vi "Test.vi"() -> ()   [LabVIEW 2021]
uses:
  Commander/Commander.lvclass
  C:/Program Files (x86)/Hyper State Machine Framework/SSW_Hyper_State_Machine.lvlibp/State_Machine_Class/Main_State_Machine/Hyper_State_Machine.lvclass
  Common_State/Common_State.lvclass
  Image_Acquisition/Image_Acquisition.lvclass
  Motion_Control/Motion_Control.lvclass
  Data_Logging/Data_Logging.lvclass
  DIO/DIO.lvclass
  C:/Program Files (x86)/Hyper State Machine Framework/SSW_Hyper_State_Machine.lvlibp/State_Machine_Class/State_Machine_Module.llb/State Machine.ctl
  C:/Program Files (x86)/Hyper State Machine Framework/SSW_Hyper_State_Machine.lvlibp/State_Machine_Class/State_Machine_Module.llb/Lock_Unlock.ctl
  C:/Program Files (x86)/Hyper State Machine Framework/SSW_Hyper_State_Machine.lvlibp/State_Machine_Class/State_Machine_Module.llb/Iterval.ctl
  C:/Program Files (x86)/Hyper State Machine Framework/SSW_Hyper_State_Machine.lvlibp/State_Machine_Class/State_Machine_Module.llb/Time_Out.ctl
  <vilib>/numeric/Random Number (Range) DBL.vi
  <vilib>/Utility/High Resolution Relative Seconds.vi
  C:/Program Files (x86)/Hyper State Machine Framework/SSW_Hyper_State_Machine.lvlibp
panel:
  out "Activate":bool
  out "Lamp":bool
  out "Current_Pos":dbl caption="mm"
  in  "EMO":bool
  out "Product ID":string
  in  "Activate_Code(Blank for 30 min Trial)":string
  out "Heart_Rate":bool
  out "Heart rate(s)":dbl format="%#_6p"
  out "Execute rate(Hz)":dbl format="%#_6p"
  out "Base Class_Time_Act":bool
  out "Base Class_Elapsed Time(s)":dbl format="%#_6p"
  out "Base Class":bool=TRUE
  out "Base Class_Remaining(s)":dbl format="%#_6p"
  out "Base Class Progress":dbl(slide) scale=0.0..30.0
  in  "Base Class":dbl=30.0 max=1000.0 format="%#_13p"
  out "Base Class":string
  out "Base Class_Active":bool
  in  "Action Manager":T1(ring)
  out "Common":bool=TRUE
  out "Common_State":string
  out "Common_Time_Act":bool
  out "Common_Elapsed Time(s)":dbl format="%#_6p"
  out "Common_State Progress":dbl(slide) scale=0.0..3.0
  in  "Common_State_Interval":dbl=3.0 max=1000.0 format="%#_13p"
  out "Common_State_Active":bool
  out "Common_State_Remaining(s)":dbl format="%#_6p"
  out "Data Logging Progress":dbl(slide) scale=0.0..0.01
  out "DIO Progress":dbl(slide) scale=0.0..0.01
  out "Motion Control Progress":dbl(slide) scale=0.0..0.05
  out "Image Acquisition Progress":dbl(slide) scale=0.0..0.01
  out "Commander Progress":dbl(slide)=-1.0 scale=0.0..1.0
  out "Data_Logging":bool=TRUE
  out "Data Logging":string
  out "Data_Logging_Time_Act":bool
  out "Data_Logging_Elapsed Time(s)":dbl format="%#_6p"
  out "DIO":bool=TRUE
  out "DIO":string
  out "DIO_Time_Act":bool
  out "DIO_Elapsed Time(s)":dbl format="%#_6p"
  out "Motion_Control":bool=TRUE
  out "Motion_Control":string
  out "Motion_Control_Time_Act":bool
  out "Motion_Control_Elapsed Time(s)":dbl format="%#_6p"
  in  "Data Logging":dbl max=1000.0 format="%#_13p"
  out "Data Logging_Active":bool
  out "Data Logging_Remaining(s)":dbl format="%#_6p"
  in  "DIO_Interval":dbl=0.01 max=1000.0 format="%#_13p"
  in  "Motion_Control_Interval":dbl=0.05 max=1000.0 format="%#_13p"
  out "Motion Control_Act":bool
  out "DIO_Act":bool
  out "DIO_Remaining(s)":dbl format="%#_6p"
  out "Motion_Control_Remaining(s)":dbl format="%#_6p"
  in  "Image Acquisition_Interval":dbl=0.01 max=1000.0 format="%#_13p"
  in  "Commander_Interval":dbl max=1000.0 format="%#_13p"
  in  "System_Wait_Time":dbl=0.01 format="%#_13p"
  out "Commander_Active":bool
  out "Image Acquisition_Act":bool
  out "Image Acquisition_Remaining(s)":dbl format="%#_6p"
  out "Commander_Remaining(s)":dbl format="%#_6p"
  out "Image Acquisition":bool=TRUE
  out "Image Acquisition":string
  out "Commander":bool=TRUE
  out "Image Acquisition_Time_Act":bool
  out "Image Acquisition_Elapsed Time(s)":dbl format="%#_6p"
  out "Commander":string
  out "State1_Time_Act":bool
  out "Commander_Elapsed Time(s)":dbl format="%#_6p"
  in  "Stop":bool
  # "Note : Each State is Waiting Until Commader State Finished on \"Interval_Delay\" and then Unlock"
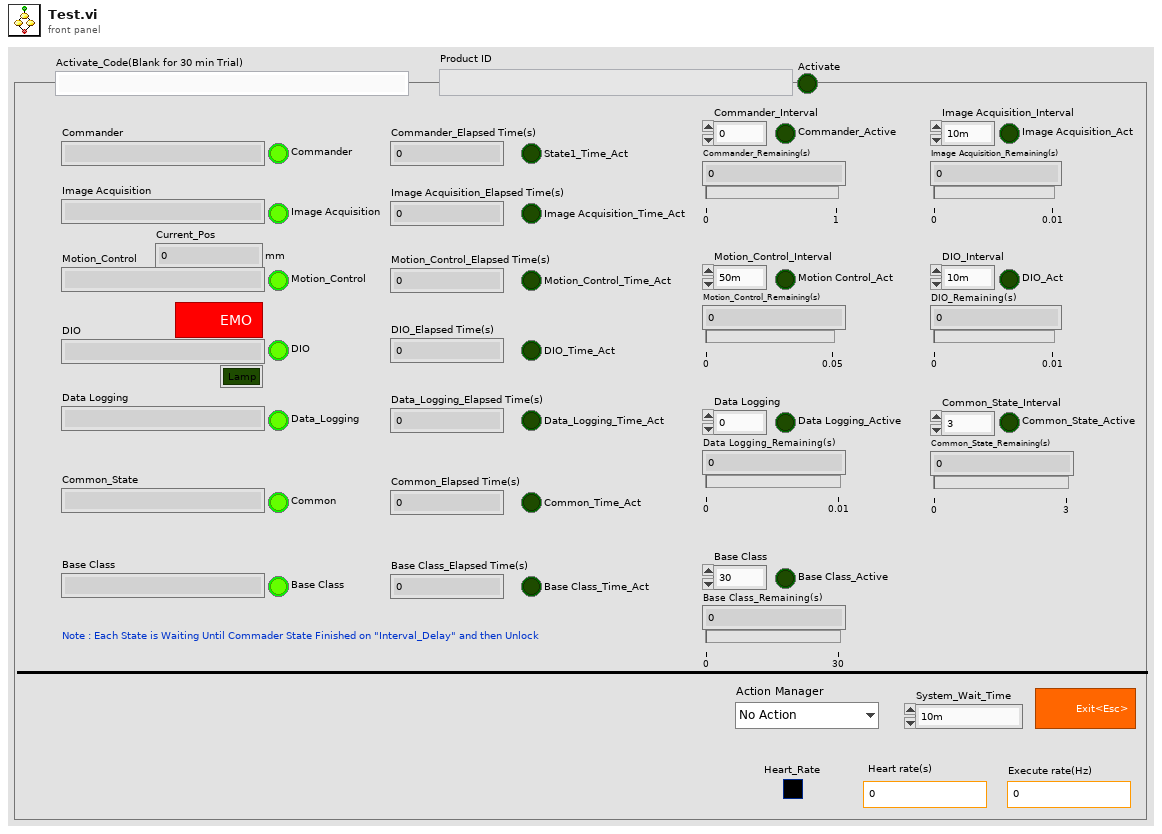
[diagram p1: front panel]
types:
  T1 = enum16{"No Action", "Init", "Lock", "Unlock", "Release"}
  T2 = typedef "SSW_Hyper_State_Machine.lvlibp/State Machine.ctl" = cluster{"Command":string, "Data":variant}
  T3 = typedef "SSW_Hyper_State_Machine.lvlibp/Time_Out.ctl" = cluster{"Enable(True)":bool, "Time Out_State Name":string, "Time Target (1s)":dbl, "Time Out_Reply Message_State":string}
  T4 = typedef "SSW_Hyper_State_Machine.lvlibp/Lock_Unlock.ctl" = cluster{"Action_Mode (Get)":enum16{"Set", "Get"}, "Action_Set (False)":bool, "State_In (Wait)":string}
  T5 = typedef "SSW_Hyper_State_Machine.lvlibp/Iterval.ctl" = cluster{"Delay(s)":dbl, "State (Interval_Delay)":string}
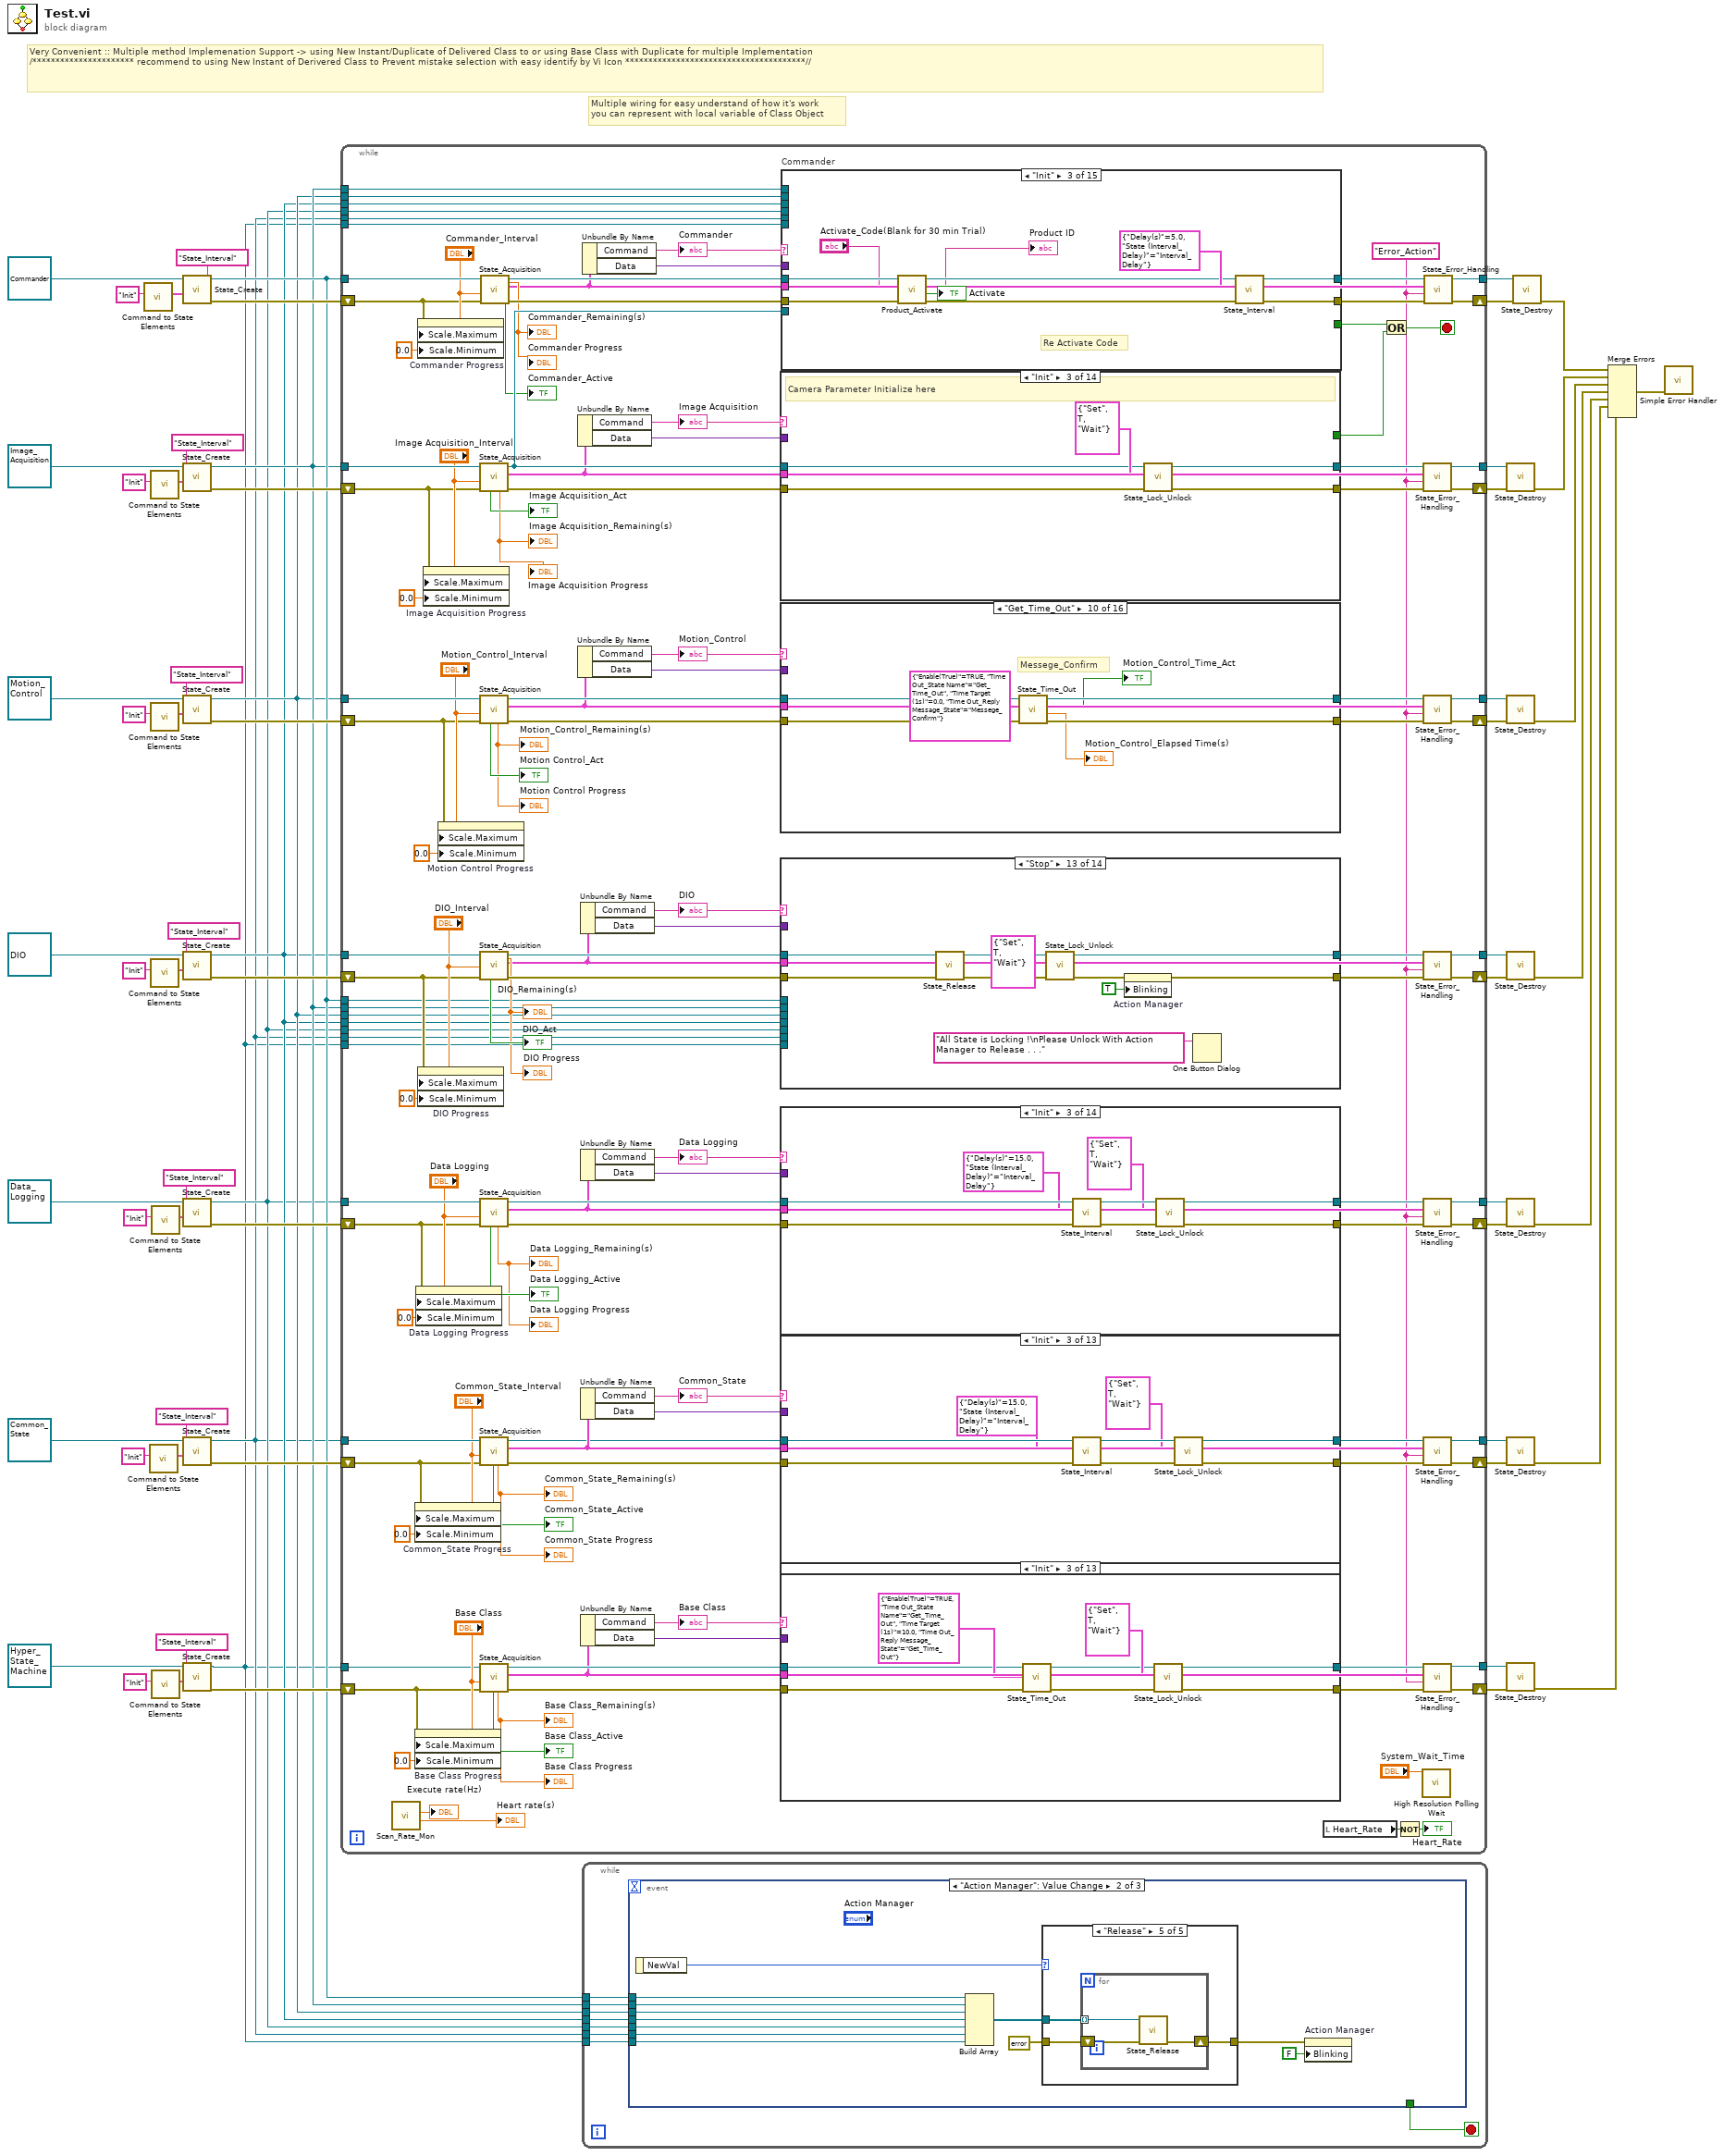
[diagram p0: block diagram]
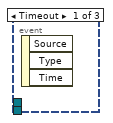
[diagram p2: hidden frame]
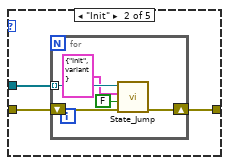
[diagram p4: hidden frame]
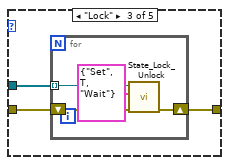
[diagram p5: hidden frame]
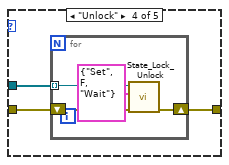
[diagram p6: hidden frame]
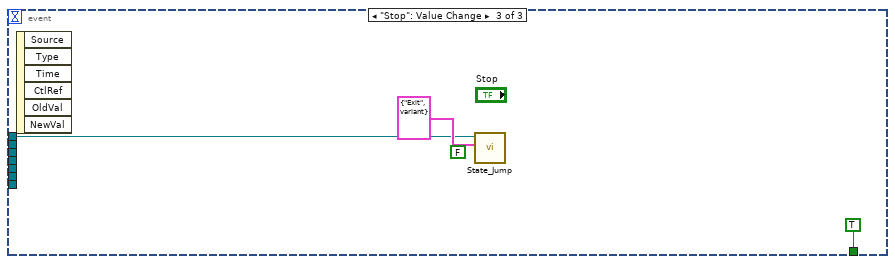
[diagram p7: hidden frame]
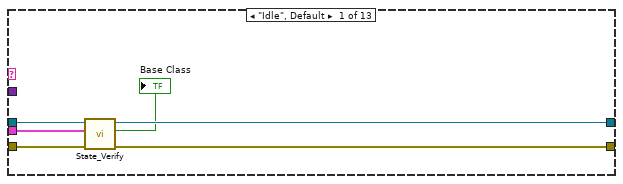
[diagram p8: hidden frame]
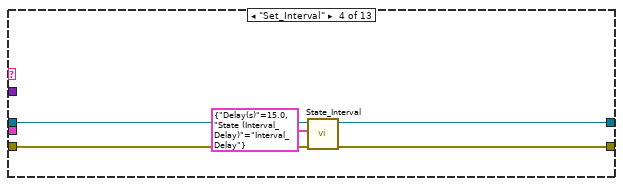
[diagram p10: hidden frame]
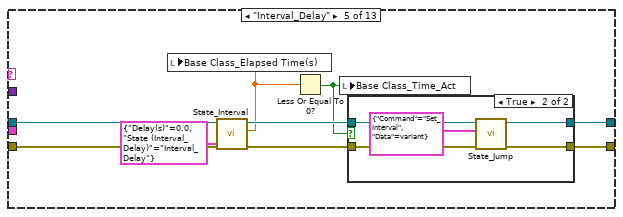
[diagram p11: hidden frame]
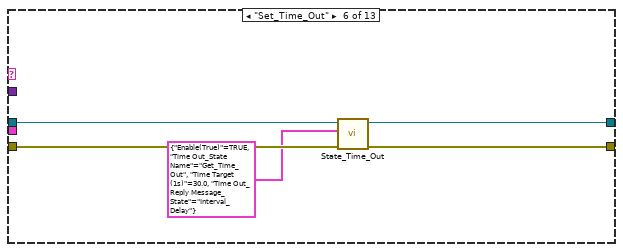
[diagram p13: hidden frame]
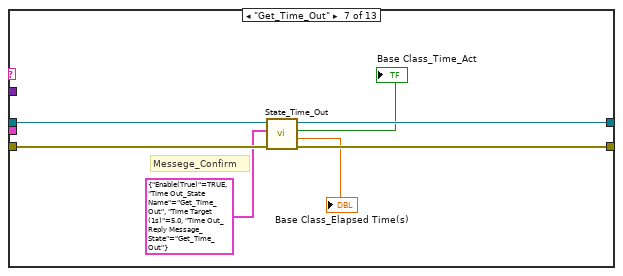
[diagram p14: hidden frame]
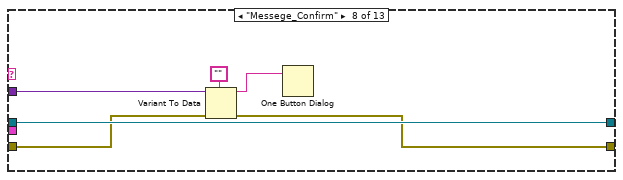
[diagram p15: hidden frame]
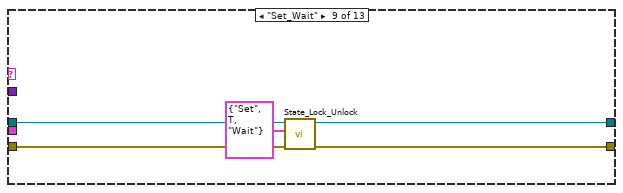
[diagram p16: hidden frame]
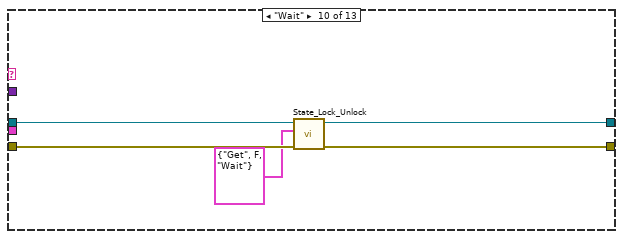
[diagram p17: hidden frame]
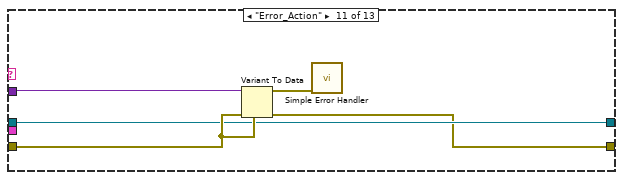
[diagram p18: hidden frame]
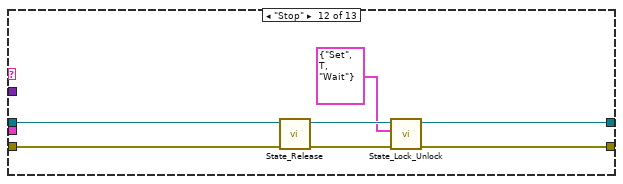
[diagram p19: hidden frame]
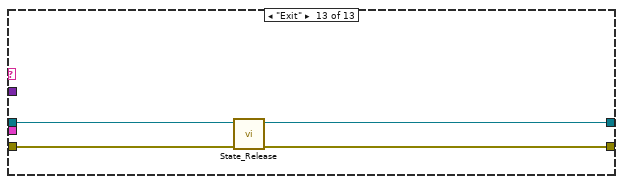
[diagram p20: hidden frame]
diagram:
  # "Multiple wiring for easy understand of how it's work\nyou can represent with local variable of Class Object"
  # "Very Convenient :: Multiple method Implemenation Support -> using New Instant/Duplicate of Delivered Class to or using Base Class with Duplicate for multiple Implementation\n/********************** recommend to using New Instant of Derivered Class to Prevent mistake selection with easy identify by Vi Icon ***************************************//"
  n1 = call "Command to State Elements.vi"("Command"="Init") -> ("Command to State Elements"=w25:T2)  [unwired: 10 in]
  n2 = call "Command to State Elements.vi"("Command"="Init") -> ("Command to State Elements"=w17:T2)  [unwired: 10 in]
  n3 = call "Command to State Elements.vi"("Command"="Init") -> ("Command to State Elements"=w27:T2)  [unwired: 10 in]
  n4 = call "Command to State Elements.vi"("Command"="Init") -> ("Command to State Elements"=w23:T2)  [unwired: 10 in]
  n5 = call "Command to State Elements.vi"("Command"="Init") -> ("Command to State Elements"=w21:T2)  [unwired: 10 in]
  n6 = call "Command to State Elements.vi"("Command"="Init") -> ("Command to State Elements"=w19:T2)  [unwired: 10 in]
  n7 = call "Command to State Elements.vi"("Command"="Init") -> ("Command to State Elements"=w15:T2)  [unwired: 10 in]
  n8 = call-dynamic "State_Create.vi"("Init_State(Option)"=w25, "State_Interval_Name"="State_Interval" ("Core_Interval_Name(State_Interval)"), "State_Machine_Class in"=refnum<class "Commander.lvclass"> refnum ("Commander.lvclass")) -> ("error out"=w64:errorcluster, "State_Machine_Class out"=w7:refnum<class "Commander.lvclass">)  [unwired: 6 in, 1 out]
  n9 = call-dynamic "State_Create.vi"("Init_State(Option)"=w27, "State_Interval_Name"="State_Interval" ("Core_Interval_Name(State_Interval)"), "State_Machine_Class in"=refnum<class "Image_Acquisition.lvclass"> refnum ("Image_Acquisition.lvclass")) -> ("error out"=w61:errorcluster, "State_Machine_Class out"=w6:refnum<class "Image_Acquisition.lvclass">)  [unwired: 6 in, 1 out]
  n10 = call-dynamic "State_Create.vi"("Init_State(Option)"=w23, "State_Interval_Name"="State_Interval" ("Core_Interval_Name(State_Interval)"), "State_Machine_Class in"=refnum<class "Motion_Control.lvclass"> refnum ("Motion_Control.lvclass")) -> ("error out"=w49:errorcluster, "State_Machine_Class out"=w5:refnum<class "Motion_Control.lvclass">)  [unwired: 6 in, 1 out]
  n11 = call-dynamic "State_Create.vi"("Init_State(Option)"=w21, "State_Interval_Name"="State_Interval" ("Core_Interval_Name(State_Interval)"), "State_Machine_Class in"=refnum<class "DIO.lvclass"> refnum ("DIO.lvclass")) -> ("error out"=w47:errorcluster, "State_Machine_Class out"=w4:refnum<class "DIO.lvclass">)  [unwired: 6 in, 1 out]
  n12 = call-dynamic "State_Create.vi"("Init_State(Option)"=w19, "State_Interval_Name"="State_Interval" ("Core_Interval_Name(State_Interval)"), "State_Machine_Class in"=refnum<class "Data_Logging.lvclass"> refnum ("Data_Logging.lvclass")) -> ("error out"=w43:errorcluster, "State_Machine_Class out"=w3:refnum<class "Data_Logging.lvclass">)  [unwired: 6 in, 1 out]
  n13 = call-dynamic "State_Create.vi"("Init_State(Option)"=w17, "State_Interval_Name"="State_Interval" ("Core_Interval_Name(State_Interval)"), "State_Machine_Class in"=refnum<class "Common_State.lvclass"> refnum ("Common_State.lvclass")) -> ("error out"=w38:errorcluster, "State_Machine_Class out"=w2:refnum<class "Common_State.lvclass">)  [unwired: 6 in, 1 out]
  n14 = call-dynamic "State_Create.vi"("Init_State(Option)"=w15, "State_Interval_Name"="State_Interval" ("Core_Interval_Name(State_Interval)"), "State_Machine_Class in"=refnum<class "Hyper_State_Machine.lvclass"> refnum ("SSW_Hyper_State_Machine.lvlibp:Hyper_State_Machine.lvclass")) -> ("error out"=w32:errorcluster, "State_Machine_Class out"=w1:refnum<class "Hyper_State_Machine.lvclass">)  [unwired: 6 in, 1 out]
  n15 = while {
    tunnel: w7 -> [w176]
    shift-right: [w185] -> w63
    shift-left: w64 -> [w84]
    tunnel: [w184] -> w62
    tunnel: w6 -> [w180]
    tunnel: [w179] -> w60
    shift-right: [w178] -> w59
    shift-left: w61 -> [w83]
    tunnel: [w154] -> w51
    tunnel: [w153] -> w50
    tunnel: w5 -> [w152]
    tunnel: w4 -> [w151]
    tunnel: w3 -> [w150]
    shift-right: [w149] -> w48
    shift-left: w49 -> [w82]
    tunnel: [w147] -> w45
    shift-right: [w148] -> w46
    shift-left: w47 -> [w81]
    shift-right: [w146] -> w44
    shift-left: w43 -> [w80]
    tunnel: w2 -> [w125]
    tunnel: [w124] -> w37
    shift-right: [w123] -> w36
    shift-left: w38 -> [w79]
    shift-right: [w93] -> w31
    shift-left: w32 -> [w78]
    tunnel: w1 -> [w97]
    tunnel: [w92] -> w30
    tunnel: w6 -> [w77]
    tunnel: w5 -> [w76]
    tunnel: w4 -> [w75]
    tunnel: w3 -> [w74]
    tunnel: w2 -> [w73]
    tunnel: w1 -> [w72]
    tunnel: w7 -> [w71]
    tunnel: w6 -> [w70]
    tunnel: w5 -> [w69]
    tunnel: w4 -> [w68]
    tunnel: w3 -> [w67]
    tunnel: w2 -> [w66]
    tunnel: w1 -> [w65]
    stop <- w175 stop-if-true
    w91 = "Error_Action" ("State_Error_Handling")
    n16 = call "Scan_Rate_Mon.vi"() -> ("Heart rate(s)"=→"Heart rate(s)":dbl, "Execute rate(Hz)"=→"Execute rate(Hz)":dbl)
    n17 = property on="Common_State Progress" class="Slide (strict)"(error in=w79, "Scale.Maximum"="Common_State_Interval", "Scale.Minimum"=0.0 ("Scale.Range:Minimum")) -> ()  [unwired: 1 in, 2 out]
    n18 = property on="Base Class Progress" class="Slide (strict)"(error in=w78, "Scale.Maximum"="Base Class", "Scale.Minimum"=0.0 ("Scale.Range:Minimum")) -> ()  [unwired: 1 in, 2 out]
    n19 = property on="Data Logging Progress" class="Slide (strict)"(error in=w80, "Scale.Maximum"="Data Logging", "Scale.Minimum"=0.0 ("Scale.Range:Minimum")) -> ()  [unwired: 1 in, 2 out]
    n20 = property on="Commander Progress" class="Slide (strict)"(error in=w84, "Scale.Maximum"="Commander_Interval", "Scale.Minimum"=0.0 ("Scale.Range:Minimum")) -> ()  [unwired: 1 in, 2 out]
    n21 = property on="DIO Progress" class="Slide (strict)"(error in=w81, "Scale.Maximum"="DIO_Interval", "Scale.Minimum"=0.0 ("Scale.Range:Minimum")) -> ()  [unwired: 1 in, 2 out]
    n22 = property on="Image Acquisition Progress" class="Slide (strict)"(error in=w83, "Scale.Maximum"="Image Acquisition_Interval", "Scale.Minimum"=0.0 ("Scale.Range:Minimum")) -> ()  [unwired: 1 in, 2 out]
    n23 = property on="Motion Control Progress" class="Slide (strict)"(error in=w82, "Scale.Maximum"="Motion_Control_Interval", "Scale.Minimum"=0.0 ("Scale.Range:Minimum")) -> ()  [unwired: 1 in, 2 out]
    n24 = call-dynamic "State_Acquisition.vi"("error in (no error)"=w83, "State_Interval_Time(s)"="Image Acquisition_Interval", "Main_Machine_State_Class in"=w180) -> ("error out"=w183:errorcluster, "State"=w110:T2, "Main_Machine_State_Class out"=w177:refnum<class "Image_Acquisition.lvclass">, "Remaining(ms)"=→"Image Acquisition_Remaining(s)" →"Image Acquisition Progress":dbl, "Current_State_Active"=→"Image Acquisition_Act":bool)  [unwired: 2 in, 2 out]
    n25 = call-dynamic "State_Acquisition.vi"("error in (no error)"=w82, "State_Interval_Time(s)"="Motion_Control_Interval", "Main_Machine_State_Class in"=w152) -> ("error out"=w156:errorcluster, "State"=w109:T2, "Main_Machine_State_Class out"=w157:refnum<class "Motion_Control.lvclass">, "Remaining(ms)"=→"Motion_Control_Remaining(s)" →"Motion Control Progress":dbl, "Current_State_Active"=→"Motion Control_Act":bool)  [unwired: 2 in, 2 out]
    n26 = call-dynamic "State_Acquisition.vi"("error in (no error)"=w81, "State_Interval_Time(s)"="DIO_Interval", "Main_Machine_State_Class in"=w151) -> ("error out"=w163:errorcluster, "State"=w108:T2, "Main_Machine_State_Class out"=w164:refnum<class "DIO.lvclass">, "Remaining(ms)"=→"DIO_Remaining(s)" →"DIO Progress":dbl, "Current_State_Active"=→"DIO_Act":bool)  [unwired: 2 in, 2 out]
    n27 = call-dynamic "State_Acquisition.vi"("error in (no error)"=w80, "State_Interval_Time(s)"="Data Logging", "Main_Machine_State_Class in"=w150) -> ("error out"=w165:errorcluster, "State"=w107:T2, "Main_Machine_State_Class out"=w166:refnum<class "Data_Logging.lvclass">, "Remaining(ms)"=→"Data Logging_Remaining(s)" →"Data Logging Progress":dbl, "Current_State_Active"=→"Data Logging_Active":bool)  [unwired: 2 in, 2 out]
    n28 = call-dynamic "State_Acquisition.vi"("error in (no error)"=w79, "State_Interval_Time(s)"="Common_State_Interval", "Main_Machine_State_Class in"=w125) -> ("error out"=w127:errorcluster, "State"=w106:T2, "Main_Machine_State_Class out"=w90:refnum<class "Common_State.lvclass">, "Remaining(ms)"=→"Common_State_Remaining(s)" →"Common_State Progress":dbl, "Current_State_Active"=→"Common_State_Active":bool)  [unwired: 2 in, 2 out]
    n29 = call-dynamic "State_Acquisition.vi"("error in (no error)"=w78, "State_Interval_Time(s)"="Base Class", "Main_Machine_State_Class in"=w97) -> ("error out"=w98:errorcluster, "State"=w95:T2, "Main_Machine_State_Class out"=w99:refnum<class "Hyper_State_Machine.lvclass">, "Remaining(ms)"=→"Base Class_Remaining(s)" →"Base Class Progress":dbl, "Current_State_Active"=→"Base Class_Active":bool)  [unwired: 2 in, 2 out]
    n30 = call-dynamic "State_Acquisition.vi"("error in (no error)"=w84, "State_Interval_Time(s)"="Commander_Interval", "Main_Machine_State_Class in"=w176) -> ("error out"=w187:errorcluster, "State"=w111:T2, "Main_Machine_State_Class out"=w188:refnum<class "Commander.lvclass">, "Remaining(ms)"=→"Commander_Remaining(s)" →"Commander Progress":dbl, "Current_State_Active"=→"Commander_Active":bool)  [unwired: 2 in, 2 out]
    n31 = Unbundle By Name(w110) -> ("Command"=w181:string, "Data"=w182:variant)
    "Image Acquisition" <- w181
    n32 = Unbundle By Name(w109) -> ("Command"=w140:string, "Data"=w169:variant)
    "Motion_Control" <- w140
    n33 = Unbundle By Name(w108) -> ("Command"=w141:string, "Data"=w168:variant)
    "DIO" <- w141
    n34 = Unbundle By Name(w107) -> ("Command"=w142:string, "Data"=w167:variant)
    "Data Logging" <- w142
    n35 = Unbundle By Name(w106) -> ("Command"=w120:string, "Data"=w126:variant)
    "Common_State" <- w120
    n36 = Unbundle By Name(w95) -> ("Command"=w103:string, "Data"=w100:variant)
    "Base Class" <- w103
    n37 = Unbundle By Name(w111) -> ("Command"=w191:string, "Data"=w190:variant)
    "Commander" <- w191
    n38 = case shown="\"Init\"" w181 {
      selector: w181 -> [_ _ _ w659 _ _ _ _ _ _ _ _ _ _]
      tunnel: w182 -> [_ _ _ _ _ _ _ _ w709 _ _ w723 _ _]
      tunnel: w177 -> [w650 w652 w654 w664 w669 w680 w696 w703 w707 w714 w719 w720 w731 w736]
      tunnel: w183 -> [w649 w651 w653 w663 w668 w679 w695 w702 w706 w713 w718 w722 w730 w735]
      tunnel: [w643 w652 w657 w662 w667 w675 w694 w701 w707 w712 w717 w720 w726 w734] -> w171
      tunnel: [w642 w651 w656 w661 w666 w674 w693 w700 w705 w711 w716 w721 w725 w733] -> w170
      tunnel: w110 -> [w648 _ _ _ _ _ _ _ _ _ _ _ _ _]
      tunnel: [_ _ _ _ _ _ _ _ _ _ _ _ _ TRUE] -> w174
      frame "Idle", Default {
        n39 = call-dynamic "State_Verify.vi"("error in (no error)"=w649, "State(Idle)"=w648, "State_Machine_Class in"=w650) -> ("error out"=w645:errorcluster, "Active"=→"Image Acquisition":bool, "State_Machine_Class out"=w646:refnum<class "Image_Acquisition.lvclass">)  [unwired: 6 in]
        n40 = call-dynamic "State_FIFO.vi"("error in (no error)"=w645, "State"=T2 {"Command"="Image_Acquisition", "Data"=variant}, "State_Machine_Class in"=w646) -> ("error out"=w642:errorcluster, "State_Machine_Class out"=w643:refnum<class "Image_Acquisition.lvclass">)  [unwired: 7 in]
      }
      frame "State_Interval" {
      }
      frame "Init" {
        # "Camera Parameter Initialize here"
        n41 = call-dynamic "State_Lock_Unlock.vi"("error in (no error)"=w653, "Parameter"=T4 {"Action_Mode (Get)"=enum."Set", "Action_Set (False)"=TRUE, "State_In (Wait)"="Wait"}, "State_Machine_Class in"=w654) -> ("error out"=w656:errorcluster, "State_Machine_Class out"=w657:refnum<class "Image_Acquisition.lvclass">)  [unwired: 6 in, 1 out]
      }
      frame "Image_Acquisition" {
        (unwired) T5 {"Delay(s)"=5.0, "State (Interval_Delay)"="Image_Acquisition"} ("Parameter")
        # "Simple handling with specify name"
        # "Dynamic handling Name for Waiting Demo"
        # "Image Acquisition Function Here"
        n42 = Bundle By Name(cluster=T5 {"Delay(s)"=5.0, "State (Interval_Delay)"=""} ("Parameter"), "State (Interval_Delay)"=w659) -> (w658:T5)
        n43 = call-dynamic "State_Interval.vi"("error in (no error)"=w663, "Parameter"=w658, "State_Machine_Class in"=w664) -> ("error out"=w661:errorcluster, "State_Machine_Class out"=w662:refnum<class "Image_Acquisition.lvclass">)  [unwired: 6 in, 1 out]
      }
      frame "Set_Interval" {
        n44 = call-dynamic "State_Interval.vi"("error in (no error)"=w668, "Parameter"=T5 {"Delay(s)"=15.0, "State (Interval_Delay)"="Interval_Delay"}, "State_Machine_Class in"=w669) -> ("error out"=w666:errorcluster, "State_Machine_Class out"=w667:refnum<class "Image_Acquisition.lvclass">)  [unwired: 6 in, 1 out]
      }
      frame "Interval_Delay" {
        n45 = call-dynamic "State_Interval.vi"("error in (no error)"=w679, "Parameter"=T5 {"Delay(s)"=0.0, "State (Interval_Delay)"="Interval_Delay"}, "State_Machine_Class in"=w680) -> ("error out"=w676:errorcluster, "Elapsed Time(s)"=w673:dbl, "State_Machine_Class out"=w677:refnum<class "Image_Acquisition.lvclass">)  [unwired: 6 in]
        "Image Acquisition_Elapsed Time(s)" <- w673
        n46 = Less Or Equal To 0?(x=w673) -> (x <= 0?=w678:bool)
        n47 = local write "Image Acquisition_Time_Act"(w678) -> ()
        n48 = case shown="True" w678 {
          tunnel: w677 -> [w682 w689]
          tunnel: w676 -> [w681 w688]
          tunnel: [w682 w684] -> w675
          tunnel: [w681 w683] -> w674
          tunnel: T2 {"Command"="Interval_Delay", "Data"=variant} ("State") -> [_ w690]
          tunnel: T2 {"Command"="Image_Acquisition", "Data"=variant} ("State") -> [_ w687]
          frame False {
          }
          frame True {
            n49 = call-dynamic "State_Jump.vi"("error in (no error)"=w688, "State"=w687, "State_Machine_Class in"=w689) -> ("error out"=w685:errorcluster, "State_Machine_Class out"=w686:refnum<class "Image_Acquisition.lvclass">)  [unwired: 7 in]
            n50 = call-dynamic "State_Jump.vi"("error in (no error)"=w685, "State"=w690, "State_Machine_Class in"=w686) -> ("error out"=w683:errorcluster, "State_Machine_Class out"=w684:refnum<class "Image_Acquisition.lvclass">)  [unwired: 7 in]
          }
        }
      }
      frame "Set_Time_Out" {
        n51 = call-dynamic "State_Time_Out.vi"("error in (no error)"=w695, "Parameter"=T3 {"Enable(True)"=TRUE, "Time Out_State Name"="Get_Time_Out", "Time Target (1s)"=30.0, "Time Out_Reply Message_State"="Messege_Confirm"}, "State_Machine_Class in"=w696) -> ("error out"=w693:errorcluster, "Timeout"=w692:bool, "State_Machine_Class out"=w694:refnum<class "Image_Acquisition.lvclass">)  [unwired: 5 in, 1 out]
        n52 = local write "Image Acquisition_Time_Act"(w692) -> ()
      }
      frame "Get_Time_Out" {
        # "Messege_Confirm"
        n53 = call-dynamic "State_Time_Out.vi"("error in (no error)"=w702, "Parameter"=T3 {"Enable(True)"=TRUE, "Time Out_State Name"="Get_Time_Out", "Time Target (1s)"=0.0, "Time Out_Reply Message_State"="Messege_Confirm"}, "State_Machine_Class in"=w703) -> ("error out"=w700:errorcluster, "Remaining Time (s)"=w699:dbl, "Timeout"=→"Image Acquisition_Time_Act":bool, "State_Machine_Class out"=w701:refnum<class "Image_Acquisition.lvclass">)  [unwired: 5 in]
        n54 = local write "Image Acquisition_Elapsed Time(s)"(w699) -> ()
      }
      frame "Messege_Confirm" {
        n55 = Variant To Data(error in=w706, type="", Variant=w709) -> (data=w704:string, error out=w705:errorcluster)
        n56 = One Button Dialog(message=w704) -> ()  [unwired: 1 in, 1 out]
      }
      frame "Set_Wait" {
        n57 = call-dynamic "State_Lock_Unlock.vi"("error in (no error)"=w713, "Parameter"=T4 {"Action_Mode (Get)"=enum."Set", "Action_Set (False)"=TRUE, "State_In (Wait)"="Wait"}, "State_Machine_Class in"=w714) -> ("error out"=w711:errorcluster, "State_Machine_Class out"=w712:refnum<class "Image_Acquisition.lvclass">)  [unwired: 6 in, 1 out]
      }
      frame "Wait" {
        n58 = call-dynamic "State_Lock_Unlock.vi"("error in (no error)"=w718, "Parameter"=T4 {"Action_Mode (Get)"=enum."Get", "Action_Set (False)"=FALSE, "State_In (Wait)"="Wait"}, "State_Machine_Class in"=w719) -> ("error out"=w716:errorcluster, "State_Machine_Class out"=w717:refnum<class "Image_Acquisition.lvclass">)  [unwired: 6 in, 1 out]
      }
      frame "Error_Action" {
        n59 = Variant To Data(error in=w722, type=w722, Variant=w723) -> (data=w724:errorcluster, error out=w721:errorcluster)
        n60 = call <vilib>:"Simple Error Handler.vi"("error in (no error)"=w724) -> ()  [unwired: 4 in, 5 out]
      }
      frame "Stop" {
        n61 = call-dynamic "State_Release.vi"("error in (no error)"=w730, "State_Machine_Class in"=w731) -> ("error out"=w728:errorcluster, "State_Machine_Class out"=w729:refnum<class "Image_Acquisition.lvclass">)  [unwired: 8 in]
        n62 = call-dynamic "State_Lock_Unlock.vi"("error in (no error)"=w728, "Parameter"=T4 {"Action_Mode (Get)"=enum."Set", "Action_Set (False)"=TRUE, "State_In (Wait)"="Wait"}, "State_Machine_Class in"=w729) -> ("error out"=w725:errorcluster, "State_Machine_Class out"=w726:refnum<class "Image_Acquisition.lvclass">)  [unwired: 6 in, 1 out]
      }
      frame "Exit" {
        n63 = call-dynamic "State_Release.vi"("error in (no error)"=w735, "State_Machine_Class in"=w736) -> ("error out"=w733:errorcluster, "State_Machine_Class out"=w734:refnum<class "Image_Acquisition.lvclass">)  [unwired: 8 in]
      }
    }
    n64 = case shown="\"Get_Time_Out\"" w140 {
      tunnel: w169 -> [_ _ _ _ _ _ _ _ _ _ w615 _ _ w628 _ _]
      tunnel: w157 -> [w553 w555 w560 w568 w573 w576 w581 w590 w602 w609 w613 w620 w625 w629 w637 w641]
      tunnel: w156 -> [w552 w554 w558 w567 w572 w575 w580 w589 w601 w608 w612 w619 w624 w627 w636 w640]
      tunnel: [w546 w555 w562 w565 w570 w576 w579 w586 w600 w607 w613 w618 w623 w629 w633 w639] -> w158
      tunnel: [w545 w554 w561 w564 w569 w575 w578 w585 w599 w606 w611 w617 w622 w626 w632 w638] -> w155
      tunnel: w109 -> [w551 _ _ _ _ _ _ _ _ _ _ _ _ _ _ _]
      frame "Idle", Default {
        n65 = call-dynamic "State_Verify.vi"("error in (no error)"=w552, "State(Idle)"=w551, "State_Machine_Class in"=w553) -> ("error out"=w548:errorcluster, "Active"=→"Motion_Control":bool, "State_Machine_Class out"=w549:refnum<class "Motion_Control.lvclass">)  [unwired: 6 in]
        n66 = call-dynamic "State_FIFO.vi"("error in (no error)"=w548, "State"=T2 {"Command"="Motion_Move", "Data"=variant}, "State_Machine_Class in"=w549) -> ("error out"=w545:errorcluster, "State_Machine_Class out"=w546:refnum<class "Motion_Control.lvclass">)  [unwired: 7 in]
      }
      frame "State_Interval" {
        # "Handling Motion I/O or Cirtical Task Here"
      }
      frame "Init" {
        # "Motion Parameter Initialize Here"
        n67 = call-dynamic "State_FIFO.vi"("error in (no error)"=w558, "State"=T2 {"Command"="Motion_Move", "Data"=variant}, "State_Machine_Class in"=w560) -> ("error out"=w557:errorcluster, "State_Machine_Class out"=w559:refnum<class "Motion_Control.lvclass">)  [unwired: 7 in]
        n68 = call-dynamic "State_Lock_Unlock.vi"("error in (no error)"=w557, "Parameter"=T4 {"Action_Mode (Get)"=enum."Set", "Action_Set (False)"=TRUE, "State_In (Wait)"="Wait"}, "State_Machine_Class in"=w559) -> ("error out"=w561:errorcluster, "State_Machine_Class out"=w562:refnum<class "Motion_Control.lvclass">)  [unwired: 6 in, 1 out]
      }
      frame "Motion_Move" {
        # "Motion Move Command here"
        n69 = call-dynamic "State_Jump.vi"("error in (no error)"=w567, "State"=T2 {"Command"="Motion_Request_Pos", "Data"=variant}, "State_Machine_Class in"=w568) -> ("error out"=w564:errorcluster, "State_Machine_Class out"=w565:refnum<class "Motion_Control.lvclass">)  [unwired: 7 in]
      }
      frame "Motion_Request_Pos" {
        # "Motion Query Position Command here"
        n70 = call-dynamic "State_Jump.vi"("error in (no error)"=w572, "State"=T2 {"Command"="Motion_Get_Pos", "Data"=variant}, "State_Machine_Class in"=w573) -> ("error out"=w569:errorcluster, "State_Machine_Class out"=w570:refnum<class "Motion_Control.lvclass">)  [unwired: 7 in]
      }
      frame "Motion_Get_Pos" {
        # "Motion Move Command here"
        n71 = call-poly <vilib>:"Random Number (Range).vi"() -> ("number"=→"Current_Pos":dbl)  [unwired: 11 in]
      }
      frame "Set_Interval" {
        n72 = call-dynamic "State_Interval.vi"("error in (no error)"=w580, "Parameter"=T5 {"Delay(s)"=15.0, "State (Interval_Delay)"="Interval_Delay"}, "State_Machine_Class in"=w581) -> ("error out"=w578:errorcluster, "State_Machine_Class out"=w579:refnum<class "Motion_Control.lvclass">)  [unwired: 6 in, 1 out]
      }
      frame "Interval_Delay" {
        n73 = call-dynamic "State_Interval.vi"("error in (no error)"=w589, "Parameter"=T5 {"Delay(s)"=0.0, "State (Interval_Delay)"="Interval_Delay"}, "State_Machine_Class in"=w590) -> ("error out"=w587:errorcluster, "Elapsed Time(s)"=w584:dbl, "State_Machine_Class out"=w588:refnum<class "Motion_Control.lvclass">)  [unwired: 6 in]
        n74 = local write "Motion_Control_Elapsed Time(s)"(w584) -> ()
        n75 = Less Or Equal To 0?(x=w584) -> (x <= 0?=w583:bool)
        n76 = local write "Motion_Control_Time_Act"(w583) -> ()
        n77 = case shown="True" w583 {
          tunnel: w588 -> [w592 w597]
          tunnel: w587 -> [w591 w596]
          tunnel: [w592 w595] -> w586
          tunnel: [w591 w594] -> w585
          frame False {
          }
          frame True {
            (unwired) FALSE ("State_Interval(Enable)")
            n78 = call-dynamic "State_Jump.vi"("error in (no error)"=w596, "State"=T2 {"Command"="Set_Interval", "Data"=variant}, "State_Machine_Class in"=w597) -> ("error out"=w594:errorcluster, "State_Machine_Class out"=w595:refnum<class "Motion_Control.lvclass">)  [unwired: 7 in]
          }
        }
      }
      frame "Set_Time_Out" {
        n79 = call-dynamic "State_Time_Out.vi"("error in (no error)"=w601, "Parameter"=T3 {"Enable(True)"=TRUE, "Time Out_State Name"="Get_Time_Out", "Time Target (1s)"=30.0, "Time Out_Reply Message_State"="Messege_Confirm"}, "State_Machine_Class in"=w602) -> ("error out"=w599:errorcluster, "State_Machine_Class out"=w600:refnum<class "Motion_Control.lvclass">)  [unwired: 5 in, 2 out]
      }
      frame "Get_Time_Out" {
        # "Messege_Confirm"
        n80 = call-dynamic "State_Time_Out.vi"("error in (no error)"=w608, "Parameter"=T3 {"Enable(True)"=TRUE, "Time Out_State Name"="Get_Time_Out", "Time Target (1s)"=0.0, "Time Out_Reply Message_State"="Messege_Confirm"}, "State_Machine_Class in"=w609) -> ("error out"=w606:errorcluster, "Remaining Time (s)"=→"Motion_Control_Elapsed Time(s)":dbl, "Timeout"=→"Motion_Control_Time_Act":bool, "State_Machine_Class out"=w607:refnum<class "Motion_Control.lvclass">)  [unwired: 5 in]
      }
      frame "Messege_Confirm" {
        n81 = Variant To Data(error in=w612, type="", Variant=w615) -> (data=w610:string, error out=w611:errorcluster)
        n82 = One Button Dialog(message=w610) -> ()  [unwired: 1 in, 1 out]
      }
      frame "Set_Wait" {
        n83 = call-dynamic "State_Lock_Unlock.vi"("error in (no error)"=w619, "Parameter"=T4 {"Action_Mode (Get)"=enum."Set", "Action_Set (False)"=TRUE, "State_In (Wait)"="Wait"}, "State_Machine_Class in"=w620) -> ("error out"=w617:errorcluster, "State_Machine_Class out"=w618:refnum<class "Motion_Control.lvclass">)  [unwired: 6 in, 1 out]
      }
      frame "Wait" {
        n84 = call-dynamic "State_Lock_Unlock.vi"("error in (no error)"=w624, "Parameter"=T4 {"Action_Mode (Get)"=enum."Get", "Action_Set (False)"=FALSE, "State_In (Wait)"="Wait"}, "State_Machine_Class in"=w625) -> ("error out"=w622:errorcluster, "State_Machine_Class out"=w623:refnum<class "Motion_Control.lvclass">)  [unwired: 6 in, 1 out]
      }
      frame "Error_Action" {
        n85 = Variant To Data(error in=w627, type=w627, Variant=w628) -> (data=w630:errorcluster, error out=w626:errorcluster)
        n86 = call <vilib>:"Simple Error Handler.vi"("error in (no error)"=w630) -> ()  [unwired: 4 in, 5 out]
      }
      frame "Stop" {
        n87 = call-dynamic "State_Release.vi"("error in (no error)"=w636, "State_Machine_Class in"=w637) -> ("error out"=w634:errorcluster, "State_Machine_Class out"=w635:refnum<class "Motion_Control.lvclass">)  [unwired: 8 in]
        n88 = call-dynamic "State_Lock_Unlock.vi"("error in (no error)"=w634, "Parameter"=T4 {"Action_Mode (Get)"=enum."Set", "Action_Set (False)"=TRUE, "State_In (Wait)"="Wait"}, "State_Machine_Class in"=w635) -> ("error out"=w632:errorcluster, "State_Machine_Class out"=w633:refnum<class "Motion_Control.lvclass">)  [unwired: 6 in, 1 out]
      }
      frame "Exit" {
        n89 = call-dynamic "State_Release.vi"("error in (no error)"=w640, "State_Machine_Class in"=w641) -> ("error out"=w638:errorcluster, "State_Machine_Class out"=w639:refnum<class "Motion_Control.lvclass">)  [unwired: 8 in]
      }
    }
    n90 = case shown="\"Stop\"" w141 {
      tunnel: w168 -> [_ _ _ _ _ _ _ _ w515 _ _ w528 _ _]
      tunnel: w164 -> [w445 w455 w472 w481 w488 w493 w500 w506 w513 w520 w525 w526 w540 w544]
      tunnel: w163 -> [w444 w446 w471 w480 w487 w492 w499 w505 w512 w519 w524 w529 w539 w543]
      tunnel: [w439 w455 w476 w479 w483 w491 w498 w504 w513 w518 w523 w526 w536 w542] -> w162
      tunnel: [w438 w446 w475 w478 w482 w490 w497 w503 w511 w517 w522 w527 w533 w541] -> w161
      tunnel: w108 -> [w443 _ _ _ _ _ _ _ _ _ _ _ _ _]
      tunnel: w71 -> [_ w453 _ _ _ _ _ _ _ _ _ _ _ _]
      tunnel: w70 -> [_ w452 _ _ _ _ _ _ _ _ _ _ _ _]
      tunnel: w69 -> [_ w451 _ _ _ _ _ _ _ _ _ _ _ _]
      tunnel: w68 -> [_ w450 _ _ _ _ _ _ _ _ _ _ _ _]
      tunnel: w67 -> [_ w449 _ _ _ _ _ _ _ _ _ _ _ _]
      tunnel: w66 -> [_ w448 _ _ _ _ _ _ _ _ _ _ _ _]
      tunnel: w65 -> [_ w447 _ _ _ _ _ _ _ _ _ _ _ _]
      frame "Idle", Default {
        # "Able to activate at \"Stae_Interval\""
        n91 = call-dynamic "State_Verify.vi"("error in (no error)"=w444, "State(Idle)"=w443, "State_Machine_Class in"=w445) -> ("error out"=w440:errorcluster, "Active"=→"DIO":bool, "State_Machine_Class out"=w441:refnum<class "DIO.lvclass">)  [unwired: 6 in]
        n92 = call-dynamic "State_FIFO.vi"("error in (no error)"=w440, "State"=T2 {"Command"="Lamp_Blinking", "Data"=variant}, "State_Machine_Class in"=w441) -> ("error out"=w438:errorcluster, "State_Machine_Class out"=w439:refnum<class "DIO.lvclass">)  [unwired: 7 in]
      }
      frame "State_Interval" {
        # "Able to assign to Even to handling"
        # "Simulation of Emergency Signal , Pree to try (Can not Override State Lock if in Active)"
        # "Simulation of Emergency Signal"
        # "Every Cycle Time DIO Get Data Here"
        n93 = case shown="True" "EMO" {
          tunnel: w453 -> [_ w465]
          tunnel: w452 -> [_ w464]
          tunnel: w451 -> [_ w463]
          tunnel: w450 -> [_ w462]
          tunnel: w449 -> [_ w461]
          tunnel: w448 -> [_ w460]
          tunnel: w447 -> [_ w459]
          tunnel: w446 -> [_ w456]
          frame False {
          }
          frame True {
            n94 = Build Array(w465, w464, w463, w462, w461, w460, w459) -> (w458:refnum<class "Hyper_State_Machine.lvclass">[])
            n95 = for {
              tunnel: w458 -> [w470] mode=indexing
              tunnel: T2 {"Command"="Stop", "Data"=variant} ("State") -> [w468]
              shift-right: [w466] -> _
              shift-left: w456 -> [w467]
              n96 = call-dynamic "State_Jump.vi"("error in (no error)"=w467, "State_Interval(Enable)"=FALSE, "State"=w468, "State_Machine_Class in"=w470) -> ("error out"=w466:errorcluster)  [unwired: 6 in, 1 out]
            }
          }
        }
      }
      frame "Init" {
        # "DIO Parameter Initialize here"
        n97 = call-dynamic "State_Lock_Unlock.vi"("error in (no error)"=w471, "Parameter"=T4 {"Action_Mode (Get)"=enum."Set", "Action_Set (False)"=TRUE, "State_In (Wait)"="Wait"}, "State_Machine_Class in"=w472) -> ("error out"=w475:errorcluster, "State_Machine_Class out"=w476:refnum<class "DIO.lvclass">)  [unwired: 6 in, 1 out]
        "Lamp" <- FALSE ("Lamp")
      }
      frame "Set_Interval" {
        n98 = call-dynamic "State_Interval.vi"("error in (no error)"=w480, "Parameter"=T5 {"Delay(s)"=15.0, "State (Interval_Delay)"="Interval_Delay"}, "State_Machine_Class in"=w481) -> ("error out"=w478:errorcluster, "State_Machine_Class out"=w479:refnum<class "DIO.lvclass">)  [unwired: 6 in, 1 out]
      }
      frame "Interval_Delay" {
        n99 = call-dynamic "State_Interval.vi"("error in (no error)"=w487, "Parameter"=T5 {"Delay(s)"=0.0, "State (Interval_Delay)"="Interval_Delay"}, "State_Machine_Class in"=w488) -> ("error out"=w482:errorcluster, "Elapsed Time(s)"=w486:dbl, "State_Machine_Class out"=w483:refnum<class "DIO.lvclass">)  [unwired: 6 in]
        n100 = local write "DIO_Elapsed Time(s)"(w486) -> ()
        n101 = Less Or Equal To 0?(x=w486) -> (x <= 0?=w485:bool)
        n102 = local write "DIO_Time_Act"(w485) -> ()
      }
      frame "Set_Time_Out" {
        n103 = call-dynamic "State_Time_Out.vi"("error in (no error)"=w492, "Parameter"=T3 {"Enable(True)"=TRUE, "Time Out_State Name"="Get_Time_Out", "Time Target (1s)"=30.0, "Time Out_Reply Message_State"="Messege_Confirm"}, "State_Machine_Class in"=w493) -> ("error out"=w490:errorcluster, "State_Machine_Class out"=w491:refnum<class "DIO.lvclass">)  [unwired: 5 in, 2 out]
      }
      frame "Get_Time_Out" {
        # "Messege_Confirm"
        n104 = call-dynamic "State_Time_Out.vi"("error in (no error)"=w499, "Parameter"=T3 {"Enable(True)"=TRUE, "Time Out_State Name"="Get_Time_Out", "Time Target (1s)"=0.0, "Time Out_Reply Message_State"="Messege_Confirm"}, "State_Machine_Class in"=w500) -> ("error out"=w497:errorcluster, "Remaining Time (s)"=→"DIO_Elapsed Time(s)":dbl, "Timeout"=→"DIO_Time_Act":bool, "State_Machine_Class out"=w498:refnum<class "DIO.lvclass">)  [unwired: 5 in]
      }
      frame "Lamp_Blinking" {
        n105 = call-dynamic "State_Interval.vi"("error in (no error)"=w505, "Parameter"=T5 {"Delay(s)"=0.25, "State (Interval_Delay)"="Lamp_Blinking"}, "State_Machine_Class in"=w506) -> ("error out"=w503:errorcluster, "Elapsed Time(s)"=w501:dbl, "State_Machine_Class out"=w504:refnum<class "DIO.lvclass">)  [unwired: 6 in]
        n106 = Less Or Equal To 0?(x=w501) -> (x <= 0?=w502:bool)
        n107 = case shown="True" w502 {
          frame False {
          }
          frame True {
            n108 = local read "Lamp"() -> (w509:bool)
            n109 = Not(x=w509) -> (.not. x?=w508:bool)
            n110 = local write "Lamp"(w508) -> ()
          }
        }
      }
      frame "Messege_Confirm" {
        n111 = Variant To Data(error in=w512, type="", Variant=w515) -> (data=w510:string, error out=w511:errorcluster)
        n112 = One Button Dialog(message=w510) -> ()  [unwired: 1 in, 1 out]
      }
      frame "Set_Wait" {
        n113 = call-dynamic "State_Lock_Unlock.vi"("error in (no error)"=w519, "Parameter"=T4 {"Action_Mode (Get)"=enum."Set", "Action_Set (False)"=TRUE, "State_In (Wait)"="Wait"}, "State_Machine_Class in"=w520) -> ("error out"=w517:errorcluster, "State_Machine_Class out"=w518:refnum<class "DIO.lvclass">)  [unwired: 6 in, 1 out]
      }
      frame "Wait" {
        n114 = call-dynamic "State_Lock_Unlock.vi"("error in (no error)"=w524, "Parameter"=T4 {"Action_Mode (Get)"=enum."Get", "Action_Set (False)"=FALSE, "State_In (Wait)"="Wait"}, "State_Machine_Class in"=w525) -> ("error out"=w522:errorcluster, "State_Machine_Class out"=w523:refnum<class "DIO.lvclass">)  [unwired: 6 in, 1 out]
      }
      frame "Error_Action" {
        n115 = Variant To Data(error in=w529, type=w529, Variant=w528) -> (data=w530:errorcluster, error out=w527:errorcluster)
        n116 = call <vilib>:"Simple Error Handler.vi"("error in (no error)"=w530) -> ()  [unwired: 4 in, 5 out]
      }
      frame "Stop" {
        n117 = call-dynamic "State_Release.vi"("error in (no error)"=w539, "State_Machine_Class in"=w540) -> ("error out"=w537:errorcluster, "State_Machine_Class out"=w538:refnum<class "DIO.lvclass">)  [unwired: 8 in]
        n118 = call-dynamic "State_Lock_Unlock.vi"("error in (no error)"=w537, "Parameter"=T4 {"Action_Mode (Get)"=enum."Set", "Action_Set (False)"=TRUE, "State_In (Wait)"="Wait"}, "State_Machine_Class in"=w538) -> ("error out"=w534:errorcluster, "State_Machine_Class out"=w536:refnum<class "DIO.lvclass">)  [unwired: 6 in, 1 out]
        n119 = property on="Action Manager" class="Enum (strict)"(error in=w534, "Blinking"=TRUE) -> (error out=w533:errorcluster)  [unwired: 1 in, 1 out]
        n120 = One Button Dialog(message="All State is Locking !\nPlease Unlock With Action Manager to Release . . .") -> ()  [unwired: 1 in, 1 out]
      }
      frame "Exit" {
        n121 = call-dynamic "State_Release.vi"("error in (no error)"=w543, "State_Machine_Class in"=w544) -> ("error out"=w541:errorcluster, "State_Machine_Class out"=w542:refnum<class "DIO.lvclass">)  [unwired: 8 in]
      }
    }
    n122 = case shown="\"Init\"" w142 {
      tunnel: w167 -> [_ _ _ _ _ _ _ _ w410 _ _ w423 _ _]
      tunnel: w166 -> [w359 w361 w369 w371 w376 w385 w397 w404 w408 w415 w420 w422 w432 w436]
      tunnel: w165 -> [w358 w360 w368 w370 w375 w384 w396 w403 w407 w414 w419 w424 w431 w435]
      tunnel: [w356 w361 w365 w371 w374 w381 w395 w402 w408 w413 w418 w422 w427 w434] -> w160
      tunnel: [w355 w360 w364 w370 w373 w380 w394 w401 w406 w412 w417 w421 w426 w433] -> w159
      tunnel: w107 -> [w357 _ _ _ _ _ _ _ _ _ _ _ _ _]
      frame "Idle", Default {
        n123 = call-dynamic "State_Verify.vi"("error in (no error)"=w358, "State(Idle)"=w357, "State_Machine_Class in"=w359) -> ("error out"=w355:errorcluster, "Active"=→"Data_Logging":bool, "State_Machine_Class out"=w356:refnum<class "Data_Logging.lvclass">)  [unwired: 6 in]
      }
      frame "State_Interval" {
        # "Files Monitering or Cirtical Task Handling Here"
      }
      frame "Init" {
        n124 = call-dynamic "State_Interval.vi"("error in (no error)"=w368, "Parameter"=T5 {"Delay(s)"=15.0, "State (Interval_Delay)"="Interval_Delay"}, "State_Machine_Class in"=w369) -> ("error out"=w363:errorcluster, "State_Machine_Class out"=w366:refnum<class "Data_Logging.lvclass">)  [unwired: 6 in, 1 out]
        n125 = call-dynamic "State_Lock_Unlock.vi"("error in (no error)"=w363, "Parameter"=T4 {"Action_Mode (Get)"=enum."Set", "Action_Set (False)"=TRUE, "State_In (Wait)"="Wait"}, "State_Machine_Class in"=w366) -> ("error out"=w364:errorcluster, "State_Machine_Class out"=w365:refnum<class "Data_Logging.lvclass">)  [unwired: 6 in, 1 out]
      }
      frame "Data_Logging" {
        # "Save Data Files Here"
      }
      frame "Set_Interval" {
        n126 = call-dynamic "State_Interval.vi"("error in (no error)"=w375, "Parameter"=T5 {"Delay(s)"=15.0, "State (Interval_Delay)"="Interval_Delay"}, "State_Machine_Class in"=w376) -> ("error out"=w373:errorcluster, "State_Machine_Class out"=w374:refnum<class "Data_Logging.lvclass">)  [unwired: 6 in, 1 out]
      }
      frame "Interval_Delay" {
        n127 = call-dynamic "State_Interval.vi"("error in (no error)"=w384, "Parameter"=T5 {"Delay(s)"=0.0, "State (Interval_Delay)"="Interval_Delay"}, "State_Machine_Class in"=w385) -> ("error out"=w382:errorcluster, "Elapsed Time(s)"=w379:dbl, "State_Machine_Class out"=w383:refnum<class "Data_Logging.lvclass">)  [unwired: 6 in]
        n128 = local write "Data_Logging_Elapsed Time(s)"(w379) -> ()
        n129 = Less Or Equal To 0?(x=w379) -> (x <= 0?=w378:bool)
        n130 = local write "Data_Logging_Time_Act"(w378) -> ()
        n131 = case shown="True" w378 {
          tunnel: w383 -> [w387 w392]
          tunnel: w382 -> [w386 w391]
          tunnel: [w387 w390] -> w381
          tunnel: [w386 w389] -> w380
          frame False {
          }
          frame True {
            (unwired) FALSE ("State_Interval(Enable)")
            n132 = call-dynamic "State_Jump.vi"("error in (no error)"=w391, "State"=T2 {"Command"="Set_Interval", "Data"=variant}, "State_Machine_Class in"=w392) -> ("error out"=w389:errorcluster, "State_Machine_Class out"=w390:refnum<class "Data_Logging.lvclass">)  [unwired: 7 in]
          }
        }
      }
      frame "Set_Time_Out" {
        n133 = call-dynamic "State_Time_Out.vi"("error in (no error)"=w396, "Parameter"=T3 {"Enable(True)"=TRUE, "Time Out_State Name"="Get_Time_Out", "Time Target (1s)"=30.0, "Time Out_Reply Message_State"="Interval_Delay"}, "State_Machine_Class in"=w397) -> ("error out"=w394:errorcluster, "State_Machine_Class out"=w395:refnum<class "Data_Logging.lvclass">)  [unwired: 5 in, 2 out]
      }
      frame "Get_Time_Out" {
        # "Messege_Confirm"
        n134 = call-dynamic "State_Time_Out.vi"("error in (no error)"=w403, "Parameter"=T3 {"Enable(True)"=TRUE, "Time Out_State Name"="Get_Time_Out", "Time Target (1s)"=0.0, "Time Out_Reply Message_State"="Messege_Confirm"}, "State_Machine_Class in"=w404) -> ("error out"=w401:errorcluster, "Remaining Time (s)"=→"Data_Logging_Elapsed Time(s)":dbl, "Timeout"=→"Data_Logging_Time_Act":bool, "State_Machine_Class out"=w402:refnum<class "Data_Logging.lvclass">)  [unwired: 5 in]
      }
      frame "Messege_Confirm" {
        n135 = Variant To Data(error in=w407, type="", Variant=w410) -> (data=w405:string, error out=w406:errorcluster)
        n136 = One Button Dialog(message=w405) -> ()  [unwired: 1 in, 1 out]
      }
      frame "Set_Wait" {
        n137 = call-dynamic "State_Lock_Unlock.vi"("error in (no error)"=w414, "Parameter"=T4 {"Action_Mode (Get)"=enum."Set", "Action_Set (False)"=TRUE, "State_In (Wait)"="Wait"}, "State_Machine_Class in"=w415) -> ("error out"=w412:errorcluster, "State_Machine_Class out"=w413:refnum<class "Data_Logging.lvclass">)  [unwired: 6 in, 1 out]
      }
      frame "Wait" {
        n138 = call-dynamic "State_Lock_Unlock.vi"("error in (no error)"=w419, "Parameter"=T4 {"Action_Mode (Get)"=enum."Get", "Action_Set (False)"=TRUE, "State_In (Wait)"="Wait"}, "State_Machine_Class in"=w420) -> ("error out"=w417:errorcluster, "State_Machine_Class out"=w418:refnum<class "Data_Logging.lvclass">)  [unwired: 6 in, 1 out]
      }
      frame "Error_Action" {
        n139 = Variant To Data(error in=w424, type=w424, Variant=w423) -> (data=w425:errorcluster, error out=w421:errorcluster)
        n140 = call <vilib>:"Simple Error Handler.vi"("error in (no error)"=w425) -> ()  [unwired: 4 in, 5 out]
      }
      frame "Stop" {
        n141 = call-dynamic "State_Release.vi"("error in (no error)"=w431, "State_Machine_Class in"=w432) -> ("error out"=w429:errorcluster, "State_Machine_Class out"=w430:refnum<class "Data_Logging.lvclass">)  [unwired: 8 in]
        n142 = call-dynamic "State_Lock_Unlock.vi"("error in (no error)"=w429, "Parameter"=T4 {"Action_Mode (Get)"=enum."Set", "Action_Set (False)"=TRUE, "State_In (Wait)"="Wait"}, "State_Machine_Class in"=w430) -> ("error out"=w426:errorcluster, "State_Machine_Class out"=w427:refnum<class "Data_Logging.lvclass">)  [unwired: 6 in, 1 out]
      }
      frame "Exit" {
        n143 = call-dynamic "State_Release.vi"("error in (no error)"=w435, "State_Machine_Class in"=w436) -> ("error out"=w433:errorcluster, "State_Machine_Class out"=w434:refnum<class "Data_Logging.lvclass">)  [unwired: 8 in]
      }
    }
    n144 = case shown="\"Init\"" w120 {
      tunnel: w126 -> [_ _ _ _ _ _ _ w327 _ _ w341 _ _]
      tunnel: w90 -> [w278 w280 w288 w293 w302 w314 w321 w325 w332 w337 w339 w349 w353]
      tunnel: w127 -> [w277 w279 w287 w292 w301 w313 w320 w324 w331 w336 w340 w348 w352]
      tunnel: [w275 w280 w282 w291 w298 w312 w319 w325 w330 w335 w339 w344 w351] -> w128
      tunnel: [w274 w279 w281 w290 w297 w311 w318 w323 w329 w334 w338 w343 w350] -> w129
      tunnel: w106 -> [w276 _ _ _ _ _ _ _ _ _ _ _ _]
      frame "Idle", Default {
        n145 = call-dynamic "State_Verify.vi"("error in (no error)"=w277, "State(Idle)"=w276, "State_Machine_Class in"=w278) -> ("error out"=w274:errorcluster, "Active"=→"Common":bool, "State_Machine_Class out"=w275:refnum<class "Common_State.lvclass">)  [unwired: 6 in]
      }
      frame "State_Interval" {
        # "Cirtical Task Handling Here"
      }
      frame "Init" {
        n146 = call-dynamic "State_Interval.vi"("error in (no error)"=w287, "Parameter"=T5 {"Delay(s)"=15.0, "State (Interval_Delay)"="Interval_Delay"}, "State_Machine_Class in"=w288) -> ("error out"=w284:errorcluster, "State_Machine_Class out"=w285:refnum<class "Common_State.lvclass">)  [unwired: 6 in, 1 out]
        n147 = call-dynamic "State_Lock_Unlock.vi"("error in (no error)"=w284, "Parameter"=T4 {"Action_Mode (Get)"=enum."Set", "Action_Set (False)"=TRUE, "State_In (Wait)"="Wait"}, "State_Machine_Class in"=w285) -> ("error out"=w281:errorcluster, "State_Machine_Class out"=w282:refnum<class "Common_State.lvclass">)  [unwired: 6 in, 1 out]
      }
      frame "Set_Interval" {
        n148 = call-dynamic "State_Interval.vi"("error in (no error)"=w292, "Parameter"=T5 {"Delay(s)"=15.0, "State (Interval_Delay)"="Interval_Delay"}, "State_Machine_Class in"=w293) -> ("error out"=w290:errorcluster, "State_Machine_Class out"=w291:refnum<class "Common_State.lvclass">)  [unwired: 6 in, 1 out]
      }
      frame "Interval_Delay" {
        n149 = call-dynamic "State_Interval.vi"("error in (no error)"=w301, "Parameter"=T5 {"Delay(s)"=5.0, "State (Interval_Delay)"="Interval_Delay"}, "State_Machine_Class in"=w302) -> ("error out"=w299:errorcluster, "Elapsed Time(s)"=w296:dbl, "State_Machine_Class out"=w300:refnum<class "Common_State.lvclass">)  [unwired: 6 in]
        n150 = local write "Common_Elapsed Time(s)"(w296) -> ()
        n151 = Less Or Equal To 0?(x=w296) -> (x <= 0?=w295:bool)
        n152 = local write "Common_Time_Act"(w295) -> ()
        n153 = case shown="True" w295 {
          tunnel: w300 -> [w304 w309]
          tunnel: w299 -> [w303 w308]
          tunnel: [w304 w307] -> w298
          tunnel: [w303 w306] -> w297
          frame False {
          }
          frame True {
            (unwired) FALSE ("State_Interval(Enable)")
            n154 = call-dynamic "State_Jump.vi"("error in (no error)"=w308, "State"=T2 {"Command"="Interval_Delay", "Data"=variant}, "State_Machine_Class in"=w309) -> ("error out"=w306:errorcluster, "State_Machine_Class out"=w307:refnum<class "Common_State.lvclass">)  [unwired: 7 in]
          }
        }
      }
      frame "Set_Time_Out" {
        n155 = call-dynamic "State_Time_Out.vi"("error in (no error)"=w313, "Parameter"=T3 {"Enable(True)"=TRUE, "Time Out_State Name"="Get_Time_Out", "Time Target (1s)"=30.0, "Time Out_Reply Message_State"="Interval_Delay"}, "State_Machine_Class in"=w314) -> ("error out"=w311:errorcluster, "State_Machine_Class out"=w312:refnum<class "Common_State.lvclass">)  [unwired: 5 in, 2 out]
      }
      frame "Get_Time_Out" {
        # "Messege_Confirm"
        # "Messege_Confirm"
        n156 = call-dynamic "State_Time_Out.vi"("error in (no error)"=w320, "Parameter"=T3 {"Enable(True)"=TRUE, "Time Out_State Name"="Get_Time_Out", "Time Target (1s)"=0.0, "Time Out_Reply Message_State"="Set_Interval"}, "State_Machine_Class in"=w321) -> ("error out"=w318:errorcluster, "Remaining Time (s)"=→"Common_Elapsed Time(s)":dbl, "Timeout"=→"Common_Time_Act":bool, "State_Machine_Class out"=w319:refnum<class "Common_State.lvclass">)  [unwired: 5 in]
      }
      frame "Messege_Confirm" {
        n157 = Variant To Data(error in=w324, type="", Variant=w327) -> (data=w322:string, error out=w323:errorcluster)
        n158 = One Button Dialog(message=w322) -> ()  [unwired: 1 in, 1 out]
      }
      frame "Set_Wait" {
        n159 = call-dynamic "State_Lock_Unlock.vi"("error in (no error)"=w331, "Parameter"=T4 {"Action_Mode (Get)"=enum."Set", "Action_Set (False)"=TRUE, "State_In (Wait)"="Wait"}, "State_Machine_Class in"=w332) -> ("error out"=w329:errorcluster, "State_Machine_Class out"=w330:refnum<class "Common_State.lvclass">)  [unwired: 6 in, 1 out]
      }
      frame "Wait" {
        n160 = call-dynamic "State_Lock_Unlock.vi"("error in (no error)"=w336, "Parameter"=T4 {"Action_Mode (Get)"=enum."Get", "Action_Set (False)"=FALSE, "State_In (Wait)"="Wait"}, "State_Machine_Class in"=w337) -> ("error out"=w334:errorcluster, "State_Machine_Class out"=w335:refnum<class "Common_State.lvclass">)  [unwired: 6 in, 1 out]
      }
      frame "Error_Action" {
        n161 = Variant To Data(error in=w340, type=w340, Variant=w341) -> (data=w342:errorcluster, error out=w338:errorcluster)
        n162 = call <vilib>:"Simple Error Handler.vi"("error in (no error)"=w342) -> ()  [unwired: 4 in, 5 out]
      }
      frame "Stop" {
        n163 = call-dynamic "State_Release.vi"("error in (no error)"=w348, "State_Machine_Class in"=w349) -> ("error out"=w346:errorcluster, "State_Machine_Class out"=w347:refnum<class "Common_State.lvclass">)  [unwired: 8 in]
        n164 = call-dynamic "State_Lock_Unlock.vi"("error in (no error)"=w346, "Parameter"=T4 {"Action_Mode (Get)"=enum."Set", "Action_Set (False)"=TRUE, "State_In (Wait)"="Wait"}, "State_Machine_Class in"=w347) -> ("error out"=w343:errorcluster, "State_Machine_Class out"=w344:refnum<class "Common_State.lvclass">)  [unwired: 6 in, 1 out]
      }
      frame "Exit" {
        n165 = call-dynamic "State_Release.vi"("error in (no error)"=w352, "State_Machine_Class in"=w353) -> ("error out"=w350:errorcluster, "State_Machine_Class out"=w351:refnum<class "Common_State.lvclass">)  [unwired: 8 in]
      }
    }
    n166 = case shown="\"Init\"" w103 {
      tunnel: w100 -> [_ _ _ _ _ _ _ w246 _ _ w260 _ _]
      tunnel: w99 -> [w197 w199 w203 w212 w221 w233 w240 w244 w251 w256 w258 w268 w272]
      tunnel: w98 -> [w196 w198 w201 w211 w220 w232 w239 w243 w250 w255 w259 w267 w271]
      tunnel: [w194 w199 w207 w210 w217 w231 w238 w244 w249 w254 w258 w263 w270] -> w96
      tunnel: [w193 w198 w206 w209 w216 w230 w237 w242 w248 w253 w257 w262 w269] -> w94
      tunnel: w95 -> [w195 _ _ _ _ _ _ _ _ _ _ _ _]
      frame "Idle", Default {
        n167 = call-dynamic "State_Verify.vi"("error in (no error)"=w196, "State(Idle)"=w195, "State_Machine_Class in"=w197) -> ("error out"=w193:errorcluster, "Active"=→"Base Class":bool, "State_Machine_Class out"=w194:refnum<class "Hyper_State_Machine.lvclass">)  [unwired: 6 in]
      }
      frame "State_Interval" {
        # "Cirtical Task Handling Here"
      }
      frame "Init" {
        n168 = call-dynamic "State_Time_Out.vi"("error in (no error)"=w201, "Parameter"=T3 {"Enable(True)"=TRUE, "Time Out_State Name"="Get_Time_Out", "Time Target (1s)"=10.0, "Time Out_Reply Message_State"="Get_Time_Out"}, "State_Machine_Class in"=w203) -> ("error out"=w200:errorcluster, "State_Machine_Class out"=w202:refnum<class "Hyper_State_Machine.lvclass">)  [unwired: 5 in, 2 out]
        n169 = call-dynamic "State_Lock_Unlock.vi"("error in (no error)"=w200, "Parameter"=T4 {"Action_Mode (Get)"=enum."Set", "Action_Set (False)"=TRUE, "State_In (Wait)"="Wait"}, "State_Machine_Class in"=w202) -> ("error out"=w206:errorcluster, "State_Machine_Class out"=w207:refnum<class "Hyper_State_Machine.lvclass">)  [unwired: 6 in, 1 out]
      }
      frame "Set_Interval" {
        n170 = call-dynamic "State_Interval.vi"("error in (no error)"=w211, "Parameter"=T5 {"Delay(s)"=15.0, "State (Interval_Delay)"="Interval_Delay"}, "State_Machine_Class in"=w212) -> ("error out"=w209:errorcluster, "State_Machine_Class out"=w210:refnum<class "Hyper_State_Machine.lvclass">)  [unwired: 6 in, 1 out]
      }
      frame "Interval_Delay" {
        n171 = call-dynamic "State_Interval.vi"("error in (no error)"=w220, "Parameter"=T5 {"Delay(s)"=0.0, "State (Interval_Delay)"="Interval_Delay"}, "State_Machine_Class in"=w221) -> ("error out"=w218:errorcluster, "Elapsed Time(s)"=w215:dbl, "State_Machine_Class out"=w219:refnum<class "Hyper_State_Machine.lvclass">)  [unwired: 6 in]
        n172 = local write "Base Class_Elapsed Time(s)"(w215) -> ()
        n173 = Less Or Equal To 0?(x=w215) -> (x <= 0?=w214:bool)
        n174 = local write "Base Class_Time_Act"(w214) -> ()
        n175 = case shown="True" w214 {
          tunnel: w219 -> [w223 w228]
          tunnel: w218 -> [w222 w227]
          tunnel: [w223 w226] -> w217
          tunnel: [w222 w225] -> w216
          frame False {
          }
          frame True {
            n176 = call-dynamic "State_Jump.vi"("error in (no error)"=w227, "State"=T2 {"Command"="Set_Interval", "Data"=variant}, "State_Machine_Class in"=w228) -> ("error out"=w225:errorcluster, "State_Machine_Class out"=w226:refnum<class "Hyper_State_Machine.lvclass">)  [unwired: 7 in]
          }
        }
      }
      frame "Set_Time_Out" {
        n177 = call-dynamic "State_Time_Out.vi"("error in (no error)"=w232, "Parameter"=T3 {"Enable(True)"=TRUE, "Time Out_State Name"="Get_Time_Out", "Time Target (1s)"=30.0, "Time Out_Reply Message_State"="Interval_Delay"}, "State_Machine_Class in"=w233) -> ("error out"=w230:errorcluster, "State_Machine_Class out"=w231:refnum<class "Hyper_State_Machine.lvclass">)  [unwired: 5 in, 2 out]
      }
      frame "Get_Time_Out" {
        # "Messege_Confirm"
        n178 = call-dynamic "State_Time_Out.vi"("error in (no error)"=w239, "Parameter"=T3 {"Enable(True)"=TRUE, "Time Out_State Name"="Get_Time_Out", "Time Target (1s)"=5.0, "Time Out_Reply Message_State"="Get_Time_Out"}, "State_Machine_Class in"=w240) -> ("error out"=w237:errorcluster, "Remaining Time (s)"=→"Base Class_Elapsed Time(s)":dbl, "Timeout"=→"Base Class_Time_Act":bool, "State_Machine_Class out"=w238:refnum<class "Hyper_State_Machine.lvclass">)  [unwired: 5 in]
      }
      frame "Messege_Confirm" {
        n179 = Variant To Data(error in=w243, type="", Variant=w246) -> (data=w241:string, error out=w242:errorcluster)
        n180 = One Button Dialog(message=w241) -> ()  [unwired: 1 in, 1 out]
      }
      frame "Set_Wait" {
        n181 = call-dynamic "State_Lock_Unlock.vi"("error in (no error)"=w250, "Parameter"=T4 {"Action_Mode (Get)"=enum."Set", "Action_Set (False)"=TRUE, "State_In (Wait)"="Wait"}, "State_Machine_Class in"=w251) -> ("error out"=w248:errorcluster, "State_Machine_Class out"=w249:refnum<class "Hyper_State_Machine.lvclass">)  [unwired: 6 in, 1 out]
      }
      frame "Wait" {
        n182 = call-dynamic "State_Lock_Unlock.vi"("error in (no error)"=w255, "Parameter"=T4 {"Action_Mode (Get)"=enum."Get", "Action_Set (False)"=FALSE, "State_In (Wait)"="Wait"}, "State_Machine_Class in"=w256) -> ("error out"=w253:errorcluster, "State_Machine_Class out"=w254:refnum<class "Hyper_State_Machine.lvclass">)  [unwired: 6 in, 1 out]
      }
      frame "Error_Action" {
        n183 = Variant To Data(error in=w259, type=w259, Variant=w260) -> (data=w261:errorcluster, error out=w257:errorcluster)
        n184 = call <vilib>:"Simple Error Handler.vi"("error in (no error)"=w261) -> ()  [unwired: 4 in, 5 out]
      }
      frame "Stop" {
        n185 = call-dynamic "State_Release.vi"("error in (no error)"=w267, "State_Machine_Class in"=w268) -> ("error out"=w265:errorcluster, "State_Machine_Class out"=w266:refnum<class "Hyper_State_Machine.lvclass">)  [unwired: 8 in]
        n186 = call-dynamic "State_Lock_Unlock.vi"("error in (no error)"=w265, "Parameter"=T4 {"Action_Mode (Get)"=enum."Set", "Action_Set (False)"=TRUE, "State_In (Wait)"="Wait"}, "State_Machine_Class in"=w266) -> ("error out"=w262:errorcluster, "State_Machine_Class out"=w263:refnum<class "Hyper_State_Machine.lvclass">)  [unwired: 6 in, 1 out]
      }
      frame "Exit" {
        n187 = call-dynamic "State_Release.vi"("error in (no error)"=w271, "State_Machine_Class in"=w272) -> ("error out"=w269:errorcluster, "State_Machine_Class out"=w270:refnum<class "Hyper_State_Machine.lvclass">)  [unwired: 8 in]
      }
    }
    n188 = case "Commander" shown="\"Init\"" w191 {
      tunnel: w190 -> [_ _ _ _ _ _ _ w800 w808 _ _ _ w834 _ _]
      tunnel: w188 -> [w742 w744 w751 w759 w769 w787 w794 w798 w804 w818 w826 w830 w835 w842 w847]
      tunnel: w187 -> [w740 w743 w750 w758 w768 w786 w793 w797 w807 _ w825 w829 w831 w841 w846]
      tunnel: [w739 w744 w754 w757 w764 w785 w792 w798 w804 w818 w824 w828 w835 w838 w845] -> w112
      tunnel: [w738 w743 w753 w756 w763 w784 w791 w796 w803 w817 w823 w827 w832 w837 w844] -> w186
      tunnel: [_ _ _ _ _ _ _ _ _ _ _ _ _ _ TRUE] -> w189
      tunnel: w111 -> [w741 _ _ _ w760 _ _ _ _ _ _ _ _ _ _]
      tunnel: w177 -> [_ _ _ _ _ _ _ _ _ _ _ _ _ _ _]
      tunnel: w77 -> [_ _ _ _ _ _ _ _ _ w815 _ _ _ _ _]
      tunnel: w76 -> [_ _ _ _ _ _ _ _ _ w814 _ _ _ _ _]
      tunnel: w75 -> [_ _ _ _ _ _ _ _ _ w813 _ _ _ _ _]
      tunnel: w74 -> [_ _ _ _ _ _ _ _ _ w812 _ _ _ _ _]
      tunnel: w73 -> [_ _ _ _ _ _ _ _ _ w811 _ _ _ _ _]
      tunnel: w72 -> [_ _ _ _ _ _ _ _ _ w810 _ _ _ _ _]
      frame "Idle", Default {
        n189 = call-dynamic "State_Verify.vi"("error in (no error)"=w740, "State(Idle)"=w741, "State_Machine_Class in"=w742) -> ("error out"=w738:errorcluster, "Active"=→"Commander":bool, "State_Machine_Class out"=w739:refnum<class "Commander.lvclass">)  [unwired: 6 in]
      }
      frame "State_Interval" {
      }
      frame "Init" {
        # "Re Activate Code"
        n190 = call-dynamic "Product_Activate.vi"("error in (no error)"=w750, "Activate Code"="Activate_Code(Blank for 30 min Trial)", "Commander in"=w751) -> ("error out"=w748:errorcluster, "Activate"=→"Activate":bool, "Product ID"=→"Product ID":string, "Commander out"=w749:refnum<class "Commander.lvclass">)  [unwired: 5 in]
        n191 = call-dynamic "State_Interval.vi"("error in (no error)"=w748, "Parameter"=T5 {"Delay(s)"=5.0, "State (Interval_Delay)"="Interval_Delay"}, "State_Machine_Class in"=w749) -> ("error out"=w753:errorcluster, "State_Machine_Class out"=w754:refnum<class "Commander.lvclass">)  [unwired: 6 in, 1 out]
      }
      frame "Set_Interval" {
        n192 = call-dynamic "State_Interval.vi"("error in (no error)"=w758, "Parameter"=T5 {"Delay(s)"=3.0, "State (Interval_Delay)"="Interval_Delay"}, "State_Machine_Class in"=w759) -> ("error out"=w756:errorcluster, "State_Machine_Class out"=w757:refnum<class "Commander.lvclass">)  [unwired: 6 in, 1 out]
      }
      frame "Interval_Delay" {
        n193 = call-dynamic "State_Interval.vi"("error in (no error)"=w768, "Parameter"=T5 {"Delay(s)"=15.0, "State (Interval_Delay)"="Interval_Delay"}, "State_Machine_Class in"=w769) -> ("error out"=w765:errorcluster, "Elapsed Time(s)"=w762:dbl, "State_Machine_Class out"=w766:refnum<class "Commander.lvclass">)  [unwired: 6 in]
        "Commander_Elapsed Time(s)" <- w762
        n194 = Less Or Equal To 0?(x=w762) -> (x <= 0?=w767:bool)
        n195 = local write "State1_Time_Act"(w767) -> ()
        n196 = case shown="True" w767 {
          tunnel: w766 -> [w771 w782]
          tunnel: w765 -> [w770 w781]
          tunnel: [w771 w779] -> w764
          tunnel: [w770 w778] -> w763
          tunnel: w760 -> [_ w777]
          frame False {
          }
          frame True {
            n197 = call-dynamic "State_FIFO.vi"("error in (no error)"=w781, "State"=T2 {"Command"="Member_Release", "Data"=variant}, "State_Machine_Class in"=w782) -> ("error out"=w774:errorcluster, "State_Machine_Class out"=w776:refnum<class "Commander.lvclass">)  [unwired: 7 in]
            n198 = call-dynamic "State_FIFO.vi"("error in (no error)"=w774, "State"=T2 {"Command"="Set_Interval", "Data"=variant}, "State_Machine_Class in"=w776) -> ("error out"=w773:errorcluster, "State_Machine_Class out"=w775:refnum<class "Commander.lvclass">)  [unwired: 7 in]
            n199 = call-dynamic "State_FIFO.vi"("error in (no error)"=w773, "State"=w777, "State_Machine_Class in"=w775) -> ("error out"=w778:errorcluster, "State_Machine_Class out"=w779:refnum<class "Commander.lvclass">)  [unwired: 7 in]
          }
        }
      }
      frame "Set_Time_Out" {
        n200 = call-dynamic "State_Time_Out.vi"("error in (no error)"=w786, "Parameter"=T3 {"Enable(True)"=TRUE, "Time Out_State Name"="Get_Time_Out", "Time Target (1s)"=30.0, "Time Out_Reply Message_State"="Messege_Confirm"}, "State_Machine_Class in"=w787) -> ("error out"=w784:errorcluster, "State_Machine_Class out"=w785:refnum<class "Commander.lvclass">)  [unwired: 5 in, 2 out]
      }
      frame "Get_Time_Out" {
        n201 = call-dynamic "State_Time_Out.vi"("error in (no error)"=w793, "Parameter"=T3 {"Enable(True)"=TRUE, "Time Out_State Name"="Get_Time_Out", "Time Target (1s)"=0.0, "Time Out_Reply Message_State"="Messege_Confirm"}, "State_Machine_Class in"=w794) -> ("error out"=w791:errorcluster, "Remaining Time (s)"=w790:dbl, "Timeout"=→"State1_Time_Act":bool, "State_Machine_Class out"=w792:refnum<class "Commander.lvclass">)  [unwired: 5 in]
        n202 = local write "Commander_Elapsed Time(s)"(w790) -> ()
      }
      frame "Messege_Confirm" {
        n203 = Variant To Data(error in=w797, type="", Variant=w800) -> (data=w795:string, error out=w796:errorcluster)
        n204 = One Button Dialog(message=w795) -> ()  [unwired: 1 in, 1 out]
      }
      frame "Dynamics_Release" {
        n205 = Variant To Data(error in=w807, type=refnum<class "Hyper_State_Machine.lvclass"> refnum ("SSW_Hyper_State_Machine.lvlibp:Hyper_State_Machine.lvclass"), Variant=w808) -> (data=w806:refnum<class "Hyper_State_Machine.lvclass">, error out=w805:errorcluster)
        n206 = call-dynamic "State_Lock_Unlock.vi"("error in (no error)"=w805, "Parameter"=T4 {"Action_Mode (Get)"=enum."Set", "Action_Set (False)"=FALSE, "State_In (Wait)"="Wait"}, "State_Machine_Class in"=w806) -> ("error out"=w803:errorcluster)  [unwired: 6 in, 2 out]
      }
      frame "Member_Release" {
        n207 = Build Array(w815, w814, w813, w812, w811, w810) -> (w809:refnum<class "Hyper_State_Machine.lvclass">[])
        n208 = for {
          tunnel: [w821] -> w817
          tunnel: T4 {"Action_Mode (Get)"=enum."Set", "Action_Set (False)"=FALSE, "State_In (Wait)"="Wait"} ("Parameter") -> [w820]
          tunnel: w809 -> [w819] mode=indexing
          n209 = call-dynamic "State_Lock_Unlock.vi"("Parameter"=w820, "State_Machine_Class in"=w819) -> ("error out"=w821:errorcluster)  [unwired: 7 in, 2 out]
        }
      }
      frame "Set_Wait" {
        n210 = call-dynamic "State_Lock_Unlock.vi"("error in (no error)"=w825, "Parameter"=T4 {"Action_Mode (Get)"=enum."Set", "Action_Set (False)"=TRUE, "State_In (Wait)"="Wait"}, "State_Machine_Class in"=w826) -> ("error out"=w823:errorcluster, "State_Machine_Class out"=w824:refnum<class "Commander.lvclass">)  [unwired: 6 in, 1 out]
      }
      frame "Wait" {
        n211 = call-dynamic "State_Lock_Unlock.vi"("error in (no error)"=w829, "State_Machine_Class in"=w830) -> ("error out"=w827:errorcluster, "State_Machine_Class out"=w828:refnum<class "Commander.lvclass">)  [unwired: 7 in, 1 out]
      }
      frame "Error_Action" {
        n212 = Variant To Data(error in=w831, type=w831, Variant=w834) -> (data=w833:errorcluster, error out=w832:errorcluster)
        n213 = call <vilib>:"Simple Error Handler.vi"("error in (no error)"=w833) -> ()  [unwired: 4 in, 5 out]
      }
      frame "Stop" {
        n214 = call-dynamic "State_Release.vi"("error in (no error)"=w841, "State_Machine_Class in"=w842) -> ("error out"=w839:errorcluster, "State_Machine_Class out"=w840:refnum<class "Commander.lvclass">)  [unwired: 8 in]
        n215 = call-dynamic "State_Lock_Unlock.vi"("error in (no error)"=w839, "Parameter"=T4 {"Action_Mode (Get)"=enum."Set", "Action_Set (False)"=TRUE, "State_In (Wait)"="Wait"}, "State_Machine_Class in"=w840) -> ("error out"=w837:errorcluster, "State_Machine_Class out"=w838:refnum<class "Commander.lvclass">)  [unwired: 6 in, 1 out]
      }
      frame "Exit" {
        n216 = call-dynamic "State_Release.vi"("error in (no error)"=w846, "State_Machine_Class in"=w847) -> ("error out"=w844:errorcluster, "State_Machine_Class out"=w845:refnum<class "Commander.lvclass">)  [unwired: 8 in]
      }
    }
    n217 = local read "Heart_Rate"() -> (w88:bool)
    n218 = Or(x=w189, y=w174) -> (x .or. y?=w175:bool)
    n219 = Not(x=w88) -> (.not. x?=→"Heart_Rate":bool)
    n220 = call <vilib>:"High Resolution Polling Wait.vi"("seconds to wait"="System_Wait_Time") -> ()  [unwired: 10 in, 1 out]
    n221 = call-dynamic "State_Error_Handling.vi"("error in (no error)"=w170, "Reply_State_Name"=w91, "Handling_State(State_Acquisition)"=w110, "State_Machine_Class in"=w171) -> ("error out"=w178:errorcluster, "State_Machine_Class out"=w179:refnum<class "Image_Acquisition.lvclass">)  [unwired: 6 in]
    n222 = call-dynamic "State_Error_Handling.vi"("error in (no error)"=w155, "Reply_State_Name"=w91, "Handling_State(State_Acquisition)"=w109, "State_Machine_Class in"=w158) -> ("error out"=w149:errorcluster, "State_Machine_Class out"=w154:refnum<class "Motion_Control.lvclass">)  [unwired: 6 in]
    n223 = call-dynamic "State_Error_Handling.vi"("error in (no error)"=w161, "Reply_State_Name"=w91, "Handling_State(State_Acquisition)"=w108, "State_Machine_Class in"=w162) -> ("error out"=w148:errorcluster, "State_Machine_Class out"=w153:refnum<class "DIO.lvclass">)  [unwired: 6 in]
    n224 = call-dynamic "State_Error_Handling.vi"("error in (no error)"=w159, "Reply_State_Name"=w91, "Handling_State(State_Acquisition)"=w107, "State_Machine_Class in"=w160) -> ("error out"=w146:errorcluster, "State_Machine_Class out"=w147:refnum<class "Data_Logging.lvclass">)  [unwired: 6 in]
    n225 = call-dynamic "State_Error_Handling.vi"("error in (no error)"=w129, "Reply_State_Name"=w91, "Handling_State(State_Acquisition)"=w106, "State_Machine_Class in"=w128) -> ("error out"=w123:errorcluster, "State_Machine_Class out"=w124:refnum<class "Common_State.lvclass">)  [unwired: 6 in]
    n226 = call-dynamic "State_Error_Handling.vi"("error in (no error)"=w94, "Reply_State_Name"=w91, "Handling_State(State_Acquisition)"=w95, "State_Machine_Class in"=w96) -> ("error out"=w93:errorcluster, "State_Machine_Class out"=w92:refnum<class "Hyper_State_Machine.lvclass">)  [unwired: 6 in]
    n227 = call-dynamic "State_Error_Handling.vi"("error in (no error)"=w186, "Reply_State_Name"=w91, "Handling_State(State_Acquisition)"=w111, "State_Machine_Class in"=w112) -> ("error out"=w185:errorcluster, "State_Machine_Class out"=w184:refnum<class "Commander.lvclass">)  [unwired: 6 in]
  }
  n228 = while {
    tunnel: w7 -> [w855]
    tunnel: w6 -> [w854]
    tunnel: w5 -> [w853]
    tunnel: w4 -> [w852]
    tunnel: w3 -> [w851]
    tunnel: w2 -> [w850]
    tunnel: w1 -> [w848]
    stop <- w849 stop-if-true
    n229 = event shown="[1] \"Action Manager\": Value Change" {
      selector: _ -> [_ _ _]
      dyn-events: _ -> [_ _ _]
      timeout: _ -> [_ _ _]
      tunnel: w855 -> [_ w866 w897]
      tunnel: w854 -> [_ w865 _]
      tunnel: w853 -> [_ w864 _]
      tunnel: w852 -> [_ w863 _]
      tunnel: w851 -> [_ w862 _]
      tunnel: w850 -> [_ w861 _]
      tunnel: [_ _ TRUE] -> w849
      tunnel: w848 -> [_ w859 _]
      event Timeout {
        n230 = event-data() -> ()  [unwired: 1 in, 3 out]
      }
      event "Action Manager": Value Change {
        n231 = event-data() -> ("NewVal"=w860:T1)  [unwired: 1 in]
        n232 = Build Array(w866, w865, w864, w863, w862, w861, w859) -> (w867:refnum<class "Hyper_State_Machine.lvclass">[])
        n233 = case shown="\"Release\"" w860 {
          tunnel: w867 -> [_ w871 w879 w886 w893]
          tunnel: [w868 w869 w878 w885 w891] -> w858
          tunnel: errorcluster {"status"=FALSE, "code"=0, "source"=""} ("error out") -> [w868 w870 w877 w884 w892]
          frame "No Action", Default {
          }
          frame "Init" {
            n234 = for {
              tunnel: w871 -> [w876] mode=indexing
              shift-right: [w872] -> w869
              shift-left: w870 -> [w874]
              n235 = call-dynamic "State_Jump.vi"("error in (no error)"=w874, "State_Interval(Enable)"=FALSE, "State"=T2 {"Command"="Init", "Data"=variant}, "State_Machine_Class in"=w876) -> ("error out"=w872:errorcluster)  [unwired: 6 in, 1 out]
            }
          }
          frame "Lock" {
            n236 = for {
              tunnel: w879 -> [w883] mode=indexing
              shift-right: [w881] -> w878
              shift-left: w877 -> [w880]
              n237 = call-dynamic "State_Lock_Unlock.vi"("error in (no error)"=w880, "Parameter"=T4 {"Action_Mode (Get)"=enum."Set", "Action_Set (False)"=TRUE, "State_In (Wait)"="Wait"}, "State_Machine_Class in"=w883) -> ("error out"=w881:errorcluster)  [unwired: 6 in, 2 out]
            }
          }
          frame "Unlock" {
            n238 = for {
              tunnel: w886 -> [w890] mode=indexing
              shift-right: [w888] -> w885
              shift-left: w884 -> [w887]
              n239 = call-dynamic "State_Lock_Unlock.vi"("error in (no error)"=w887, "Parameter"=T4 {"Action_Mode (Get)"=enum."Set", "Action_Set (False)"=FALSE, "State_In (Wait)"="Wait"}, "State_Machine_Class in"=w890) -> ("error out"=w888:errorcluster)  [unwired: 6 in, 2 out]
            }
          }
          frame "Release" {
            n240 = for {
              tunnel: w893 -> [w896] mode=indexing
              shift-right: [w894] -> w891
              shift-left: w892 -> [w895]
              n241 = call-dynamic "State_Release.vi"("error in (no error)"=w895, "State_Machine_Class in"=w896) -> ("error out"=w894:errorcluster)  [unwired: 8 in, 1 out]
            }
          }
        }
        n242 = property on="Action Manager" class="Enum (strict)"(error in=w858, "Blinking"=FALSE) -> ()  [unwired: 1 in, 2 out]
      }
      event "Stop": Value Change {
        (unwired) FALSE ("State_Interval(Enable)")
        n243 = event-data() -> ()  [unwired: 1 in, 6 out]
        n244 = call-dynamic "State_Jump.vi"("State"=T2 {"Command"="Exit", "Data"=variant}, "State_Machine_Class in"=w897) -> ()  [unwired: 8 in, 2 out]
      }
    }
  }
  n245 = call-dynamic "State_Destroy.vi"("error in (no error)"=w59, "State_Machine_Class in"=w60) -> ("error out"=w57:errorcluster)  [unwired: 8 in, 1 out]
  n246 = call-dynamic "State_Destroy.vi"("error in (no error)"=w48, "State_Machine_Class in"=w51) -> ("error out"=w42:errorcluster)  [unwired: 8 in, 1 out]
  n247 = call-dynamic "State_Destroy.vi"("error in (no error)"=w46, "State_Machine_Class in"=w50) -> ("error out"=w41:errorcluster)  [unwired: 8 in, 1 out]
  n248 = call-dynamic "State_Destroy.vi"("error in (no error)"=w44, "State_Machine_Class in"=w45) -> ("error out"=w40:errorcluster)  [unwired: 8 in, 1 out]
  n249 = call-dynamic "State_Destroy.vi"("error in (no error)"=w36, "State_Machine_Class in"=w37) -> ("error out"=w35:errorcluster)  [unwired: 8 in, 1 out]
  n250 = call-dynamic "State_Destroy.vi"("error in (no error)"=w31, "State_Machine_Class in"=w30) -> ("error out"=w29:errorcluster)  [unwired: 8 in, 1 out]
  n251 = call-dynamic "State_Destroy.vi"("error in (no error)"=w63, "State_Machine_Class in"=w62) -> ("error out"=w58:errorcluster)  [unwired: 8 in, 1 out]
  n252 = Merge Errors(w58, w57, w42, w41, w40, w35, w29) -> (w56:errorcluster)
  n253 = call <vilib>:"Simple Error Handler.vi"("error in (no error)"=w56) -> ()  [unwired: 4 in, 5 out]
